vi "MPU_Stick_Read_Serial_Port.vi"(8 "error in (no error)":errorcluster, 11 "MPU_Stick_Globals":T1) -> ()   [LabVIEW 2017]
uses:
  Controls/MPU_Stick_Globals.ctl
  Controls/IMU_Configuration_References.ctl
  Controls/MP_Comp_Filter_Constants_References.ctl
  Controls/MD_Threshold_References.ctl
  Controls/MD_Type_References.ctl
  Controls/LED_Configuration_References.ctl
  Controls/Primary_References.ctl
  Controls/MPU_Stick_Queues.ctl
  Controls/MPU_Stick_Queue_Element.ctl
  Controls/MPU_Stick_Queue_Commands.ctl
  Classes/ADCP.lvclass
  Controls/MPU_Stick_Timestamped_Data.ctl
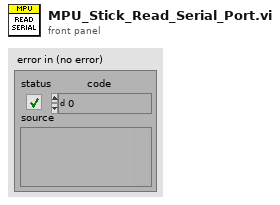
[diagram p1: front panel]
types:
  T1 = typedef "MPU_Stick_Globals.ctl" = cluster{"IMU_configuration_references":T2, "MP_Comp_Filter_Constants_References":T3, "MD_Threshold_References":T4, "MD_Type_References":T5, "LED_Configuration_References":T6, "Primary_references":T7, "MPU_Stick_Queues":T8, "ADCP":refnum<vi>}
  T2 = typedef "IMU_Configuration_References.ctl" = cluster{"Get all IMU configurations":refnum<vi>, "Set all IMU configurations":refnum<vi>, "Get sampling frequency":refnum<vi>, "Set sampling frequency":refnum<vi>, "Get calibration point count":refnum<vi>, "Set calibration point count":refnum<vi>, "Get calibration interval":refnum<vi>, "Set calibration interval":refnum<vi>, "Get Gyroscope bandwidth":refnum<vi>, "Set Gyroscope bandwidth":refnum<vi>, "Get Gyroscope F.S. Value":refnum<vi>, "Set Gyroscope F.S. Value":refnum<vi>, "Get Accelerometer bandwidth":refnum<vi>, "Set Accelerometer bandwidth":refnum<vi>, "Get Accelerometer F.S. Value":refnum<vi>, "Set Accelerometer F.S. Value":refnum<vi>, "Sampling frequency (Hz)":refnum<vi>, "Calibration point count":refnum<vi>, "Calibration interval (ms)":refnum<vi>, "IMU Gyroscope bandwidth":refnum<vi>, "IMU Gyroscope F.S. value":refnum<vi>, "IMU Accelerometer bandwidth":refnum<vi>, "IMU Accelerometer F.S. value":refnum<vi>}
  T3 = typedef "MP_Comp_Filter_Constants_References.ctl" = cluster{"Set pitch filter constant":refnum<vi>, "Get pitch filter constant":refnum<vi>, "Set roll filter constant":refnum<vi>, "Get roll filter constant":refnum<vi>, "Pitch filter constant":refnum<vi>, "Roll filter constant":refnum<vi>}
  T4 = typedef "MD_Threshold_References.ctl" = cluster{"Yaw threshold (U)":refnum<vi>, "Yaw threshold (L)":refnum<vi>, "Pitch threshold (U)":refnum<vi>, "Pitch. threshold (L)":refnum<vi>, "Roll threshold (U)":refnum<vi>, "Roll threshold (L)":refnum<vi>, "Z gyro. threshold (U)":refnum<vi>, "Z gyro. threshold (L)":refnum<vi>, "Y gyro. threshold (U)":refnum<vi>, "Y gyro. threshold (L)":refnum<vi>, "X gyro. threshold (U)":refnum<vi>, "X gyro. threshold (L)":refnum<vi>, "Z accel. threshold (U)":refnum<vi>, "Z accel. threshold (L)":refnum<vi>, "Y accel. threshold (U)":refnum<vi>, "Y accel. threshold (L)":refnum<vi>, "X accel. threshold (U)":refnum<vi>, "X accel. threshold (L)":refnum<vi>, "Set all Motion detection threshold configurations":refnum<vi>, "Get yaw threshold (upper)":refnum<vi>, "Get yaw threshold (lower)":refnum<vi>, "Get pitch threshold (upper)":refnum<vi>, "Get pitch threshold (lower)":refnum<vi>, "Get roll threshold (upper)":refnum<vi>, "Get roll threshold (lower)":refnum<vi>, "Get Z gyro threshold (upper)":refnum<vi>, "Get Z gyro threshold (lower)":refnum<vi>, "Get Y gyro threshold (upper)":refnum<vi>, "Get Y gyro threshold (lower)":refnum<vi>, "Get X gyro threshold (upper)":refnum<vi>, "Get X gyro threshold (lower)":refnum<vi>, "Get Z accel threshold (upper)":refnum<vi>, "Get Z accel threshold (lower)":refnum<vi>, "Get Y accel threshold (upper)":refnum<vi>, "Get Y accel threshold (lower)":refnum<vi>, "Get X accel threshold (upper)":refnum<vi>, "Get X accel threshold (lower)":refnum<vi>, "Get all Motion detection threshold configurations":refnum<vi>, "Set yaw threshold (upper)":refnum<vi>, "Set yaw threshold (lower)":refnum<vi>, "Set pitch threshold (upper)":refnum<vi>, "Set pitch threshold (lower)":refnum<vi>, "Set roll threshold (upper)":refnum<vi>, "Set roll threshold (lower)":refnum<vi>, "Set Z gyro threshold (upper)":refnum<vi>, "Set Z gyro threshold (lower)":refnum<vi>, "Set Y gyro threshold (upper)":refnum<vi>, "Set Y gyro threshold (lower)":refnum<vi>, "Set X gyro threshold (upper)":refnum<vi>, "Set X gyro threshold (lower)":refnum<vi>, "Set Z accel threshold (upper)":refnum<vi>, "Set Z accel threshold (lower)":refnum<vi>, "Set Y accel threshold (upper)":refnum<vi>, "Set Y accel threshold (lower)":refnum<vi>, "Set X accel threshold (upper)":refnum<vi>, "Set X accel threshold (lower)":refnum<vi>}
  T5 = typedef "MD_Type_References.ctl" = cluster{"Yaw threshold type":refnum<vi>, "Pitch threshold type":refnum<vi>, "Roll threshold type":refnum<vi>, "Z gyro threshold type":refnum<vi>, "Y gyro threshold type":refnum<vi>, "X gyro threshold type":refnum<vi>, "Z accel threshold type":refnum<vi>, "Y accel threshold type":refnum<vi>, "X accel threshold type":refnum<vi>, "Set all Motion detection type configurations":refnum<vi>, "Get all Motion detection type configurations":refnum<vi>, "Set yaw threshold type":refnum<vi>, "Get yaw threshold type":refnum<vi>, "Set pitch threshold type":refnum<vi>, "Get pitch threshold type":refnum<vi>, "Set roll threshold type":refnum<vi>, "Get roll threshold type":refnum<vi>, "Set Z gyroscope threshold type":refnum<vi>, "Get Z gyroscope threshold type":refnum<vi>, "Set Y gyroscope threshold type":refnum<vi>, "Get Y gyroscope threshold type":refnum<vi>, "Set X gyroscope threshold type":refnum<vi>, "Get X gyroscope threshold type":refnum<vi>, "Set Z accel threshold type":refnum<vi>, "Get Z accel threshold type":refnum<vi>, "Set Y accel threshold type":refnum<vi>, "Get Y accel threshold type":refnum<vi>, "Get X accel threshold type":refnum<vi>, "Set X accel threshold type":refnum<vi>}
  T6 = typedef "LED_Configuration_References.ctl" = cluster{"Get all LED configurations":refnum<vi>, "Set all LED configurations":refnum<vi>, "Get LED3 configuration":refnum<vi>, "Set LED3 configuration":refnum<vi>, "Get LED2 configuration":refnum<vi>, "Set LED2 configuration":refnum<vi>, "Get LED1 configuration":refnum<vi>, "Set LED1 configuration":refnum<vi>, "LED3 Configuration":refnum<vi>, "LED2 Configuration":refnum<vi>, "LED1 Configuration":refnum<vi>}
  T7 = typedef "Primary_References.ctl" = cluster{"3D View Image":refnum<vi>, "Plot":refnum<vi>, "Graph / 3D view tab control":refnum<vi>, "MP Reset":refnum<vi>, "Calibrate IMU":refnum<vi>, "Plot Parameter List":refnum<vi>, "Remove Parameter from Plot":refnum<vi>, "Add Parameter to Plot":refnum<vi>, "Parameter to monitor":refnum<vi>, "Yaw motion detection output":refnum<vi>, "Pitch motion detection output":refnum<vi>, "Roll motion detection output":refnum<vi>, "Z gyro motion detection output":refnum<vi>, "Y gyro motion detection output":refnum<vi>, "X gyro motion detection output":refnum<vi>, "Z accel motion detection output":refnum<vi>, "Y accel motion detection output":refnum<vi>, "X accel motion detection output":refnum<vi>, "Yaw angle (filter) (degrees)":refnum<vi>, "Pitch angle (filter) (degrees)":refnum<vi>, "Roll angle (filter) (degrees)":refnum<vi>, "Yaw angle (gyro) (degrees)":refnum<vi>, "Pitch angle (gyro) (degrees)":refnum<vi>, "Roll angle (gyro) (degrees)":refnum<vi>, "Yaw angle (accel) (degrees)":refnum<vi>, "Pitch angle (accel) (degrees)":refnum<vi>, "Roll angle (accel) (degrees)":refnum<vi>, "Z gyroscope reading (DPS)":refnum<vi>, "Y gyroscope reading (DPS)":refnum<vi>, "X gyroscope reading (DPS)":refnum<vi>, "Z accelerometer reading (G)":refnum<vi>, "Y accelerometer reading (G)":refnum<vi>, "X accelerometer reading (G)":refnum<vi>, "Save all config.":refnum<vi>, "Write all config.":refnum<vi>, "Read all config.":refnum<vi>, "Tab Control":refnum<vi>, "Baud Rate":refnum<vi>, "COM Port":refnum<vi>, "Time (ms)":refnum<vi>, "Value (Units)":refnum<vi>, "Exit Application":refnum<vi>, "Connect Device":refnum<vi>, "Progress Bar":refnum<vi>, "Get Range & Offset":refnum<vi>, "Range":refnum<vi>, "Offset":refnum<vi>, "Set Range & Offset":refnum<vi>, "Parameter name":refnum<vi>, "Plot time (ms)":refnum<vi>, "Plot value":refnum<vi>}
  T8 = typedef "MPU_Stick_Queues.ctl" = cluster{"UI Event Handler":refnum<queue>, "3D View Updater":refnum<queue>, "Plot Updater":refnum<queue>, "Serial Port Reader":refnum<queue>, "UI Indicators Updater":refnum<queue>}
  T9 = typedef "MPU_Stick_Queue_Commands.ctl" = enum16{"UI_Event_Exit_Application_RQST", "UI_Event_Exit_Application_ACK", "UI_Event_Connect_Device_RQST", "UI_Event_Connect_Device_ACK", "UI_Event_Disconnect_Device_RQST", "UI_Event_Disconnect_Device_ACK", "UI_Event_Read_All_Configurations_RQST", "UI_Event_Read_All_Configurations_ACK", "UI_Event_Write_All_Configurations_RQST", "UI_Event_Write_All_Configurations_ACK", "UI_Event_Save_All_Configurations_RQST", "UI_Event_Save_All_Configurations_ACK", "UI_Event_Calibrate_IMU_Sensor_RQST", "UI_Event_Calibrate_IMU_Sensor_ACK", "UI_Event_MP_Reset_RQST", "UI_Event_MP_Reset_ACK", "UI_Event_Get_Config_RQST", "UI_Event_Get_Config_ACK", "UI_Event_Set_Config_RQST", "UI_Event_Set_Config_ACK", "Read_Serial_Port_Data_Pause", "Read_Serial_Port_Data_Continue", "Read_Serial_Port_Data_Exit", "Plotter_Exit", "Plotter_Update", "Plotter_Add_Channel", "Plotter_Remove_Channel", "3D Viewer Update", "3D Viewer Exit", "UI Indicators Update", "UI Indicators Exit"}
  T10 = typedef "MPU_Stick_Queue_Element.ctl" = cluster{"Data":variant, "Command":T9}
  T11 = typedef "MPU_Stick_Timestamped_Data.ctl" = cluster{"Parameter name":string, "Time (ms)":dbl, "Value":dbl}
  T12 = typedef "ADCP.lvclass/ADCP_Packet_Info.ctl" = cluster{"Priority":enum16{"LOW", "HIGH"}, "Type":enum16{"Data", "Connection Management", "Remote Request", "Error and status", "INVALID"}, "Node ID":i32, "Frame ID":i32, "Checksum valid ?":bool, "Current time (ms)":u32}
  T13 = typedef "ADCP.lvclass/ADCP_Data_Packet_Transmit_Mode.ctl" = enum16{"Disable", "Single", "Cyclic", "Repeat"}
  T14 = cluster{"Parameters":cluster{"Parameter name":string, "Node name":string, "Node ID":u8, "Frame name":string, "Frame ID":u8, "Start bit":u32, "Bit length":u32, "Factor":dbl, "Offset":dbl, "Minimum":dbl, "Maximum":dbl, "Value":string, "Comments":string, "Data_Type":enum16{"BOOL", "UNSIGNED", "SIGNED", "FLOAT32", "ENUM"}, "Enum List":string[]}[], "Priority":enum16{"LOW", "HIGH"}, "Node name":string, "Node ID":u8, "Frame name":string, "Frame ID":u8, "Data":u32, "Raw bytes":u8[], "Processed bytes":u8[], "Tx count":i32, "Last Tx Time":u32, "Tx interval":u32, "Rx count":i32, "Last Rx Time":u32, "Rx interval":u32, "Tx Enable":bool, "Tx mode":T13, "Repeat/Cyclic Tx interval":u32, "Repeat count":u16}
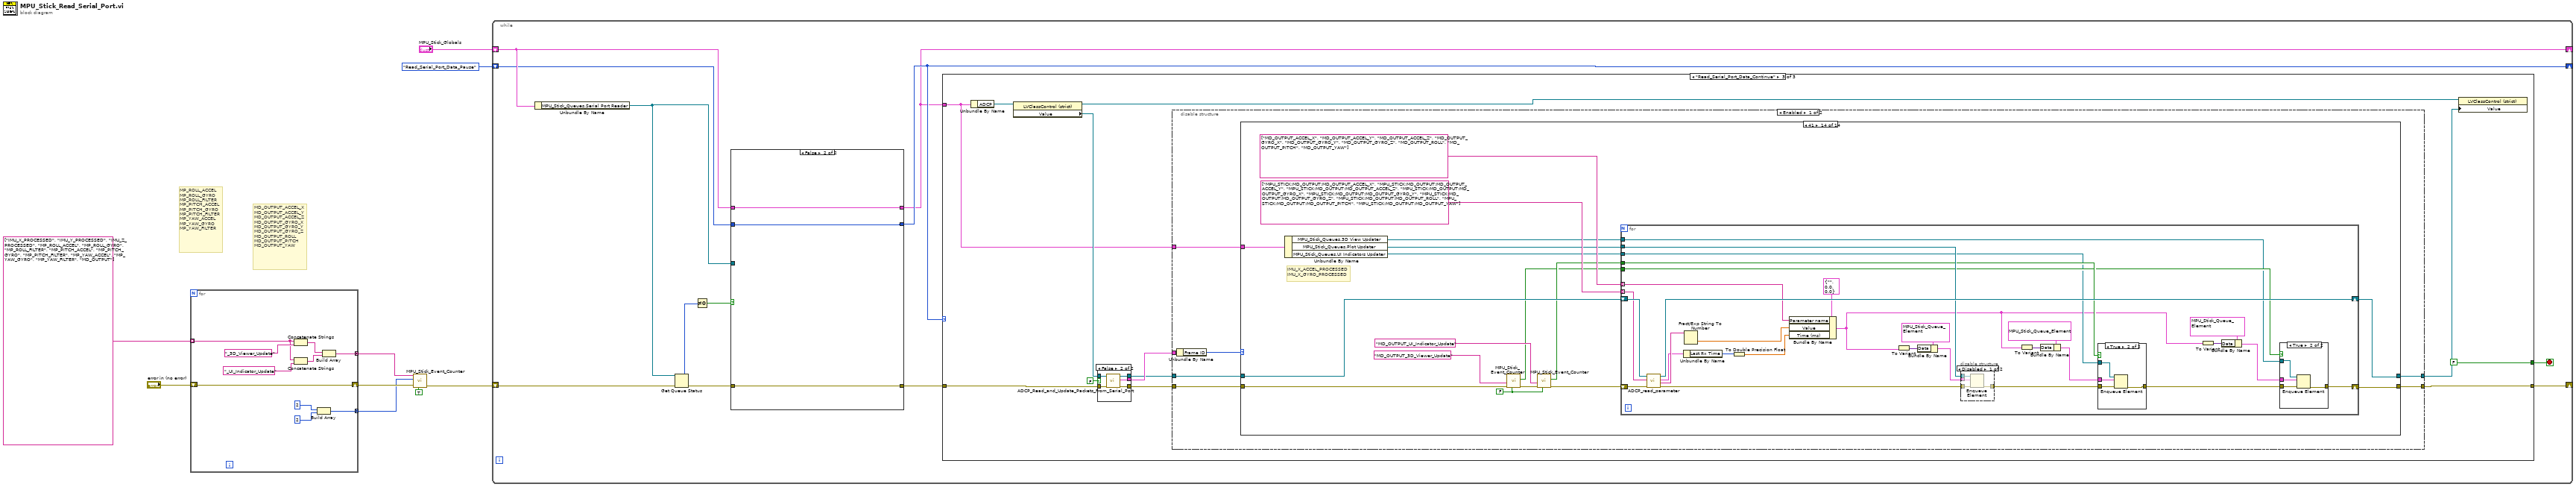
[diagram p0: block diagram]
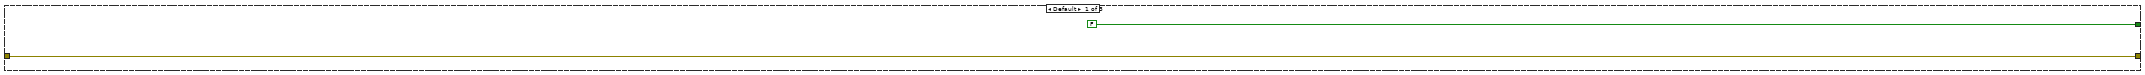
[diagram p2: hidden frame]
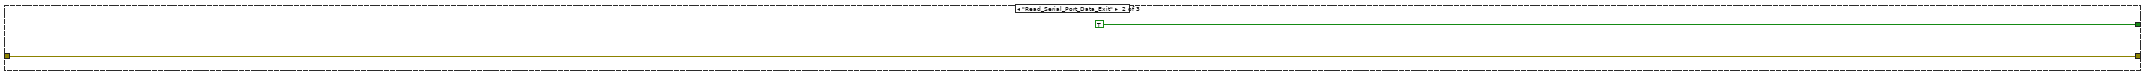
[diagram p3: hidden frame]
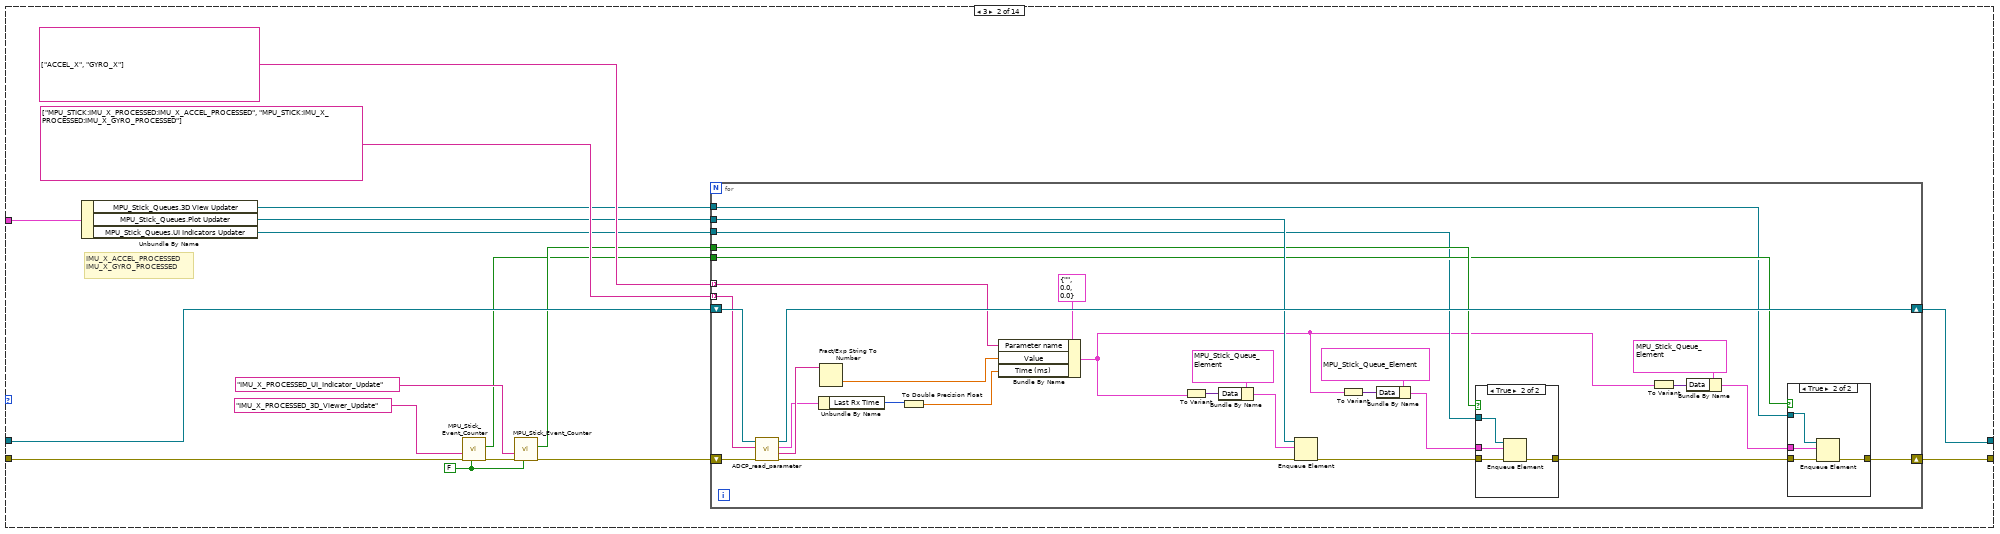
[diagram p5: hidden frame]
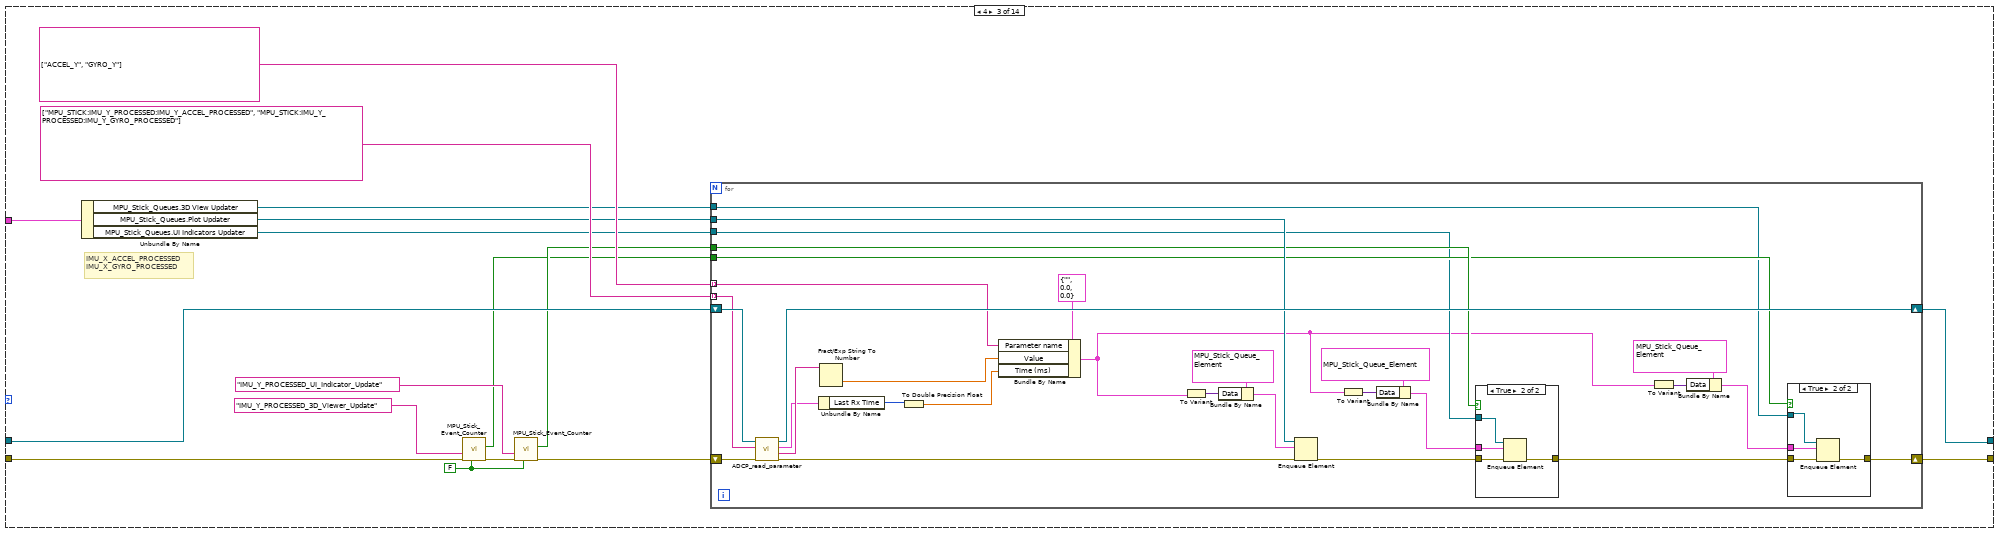
[diagram p8: hidden frame]
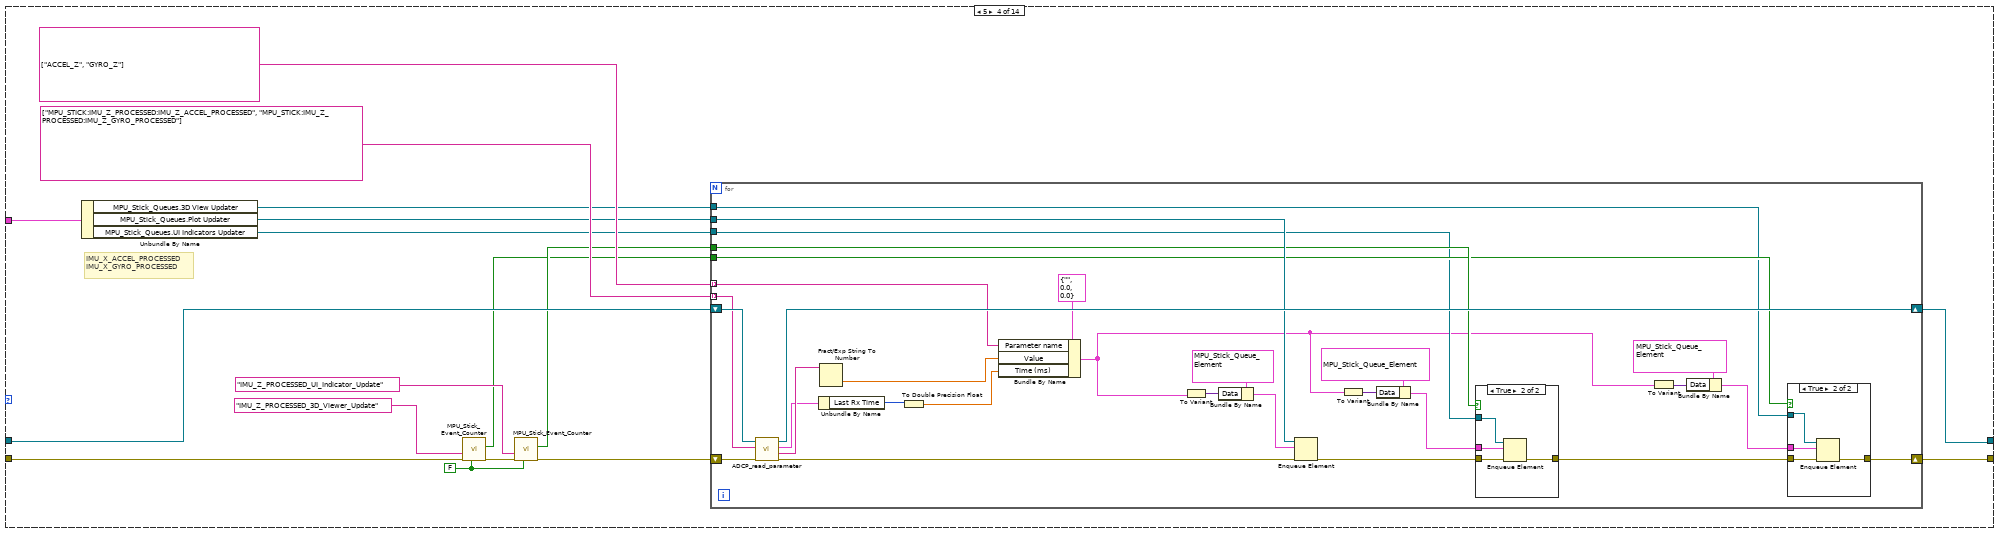
[diagram p11: hidden frame]
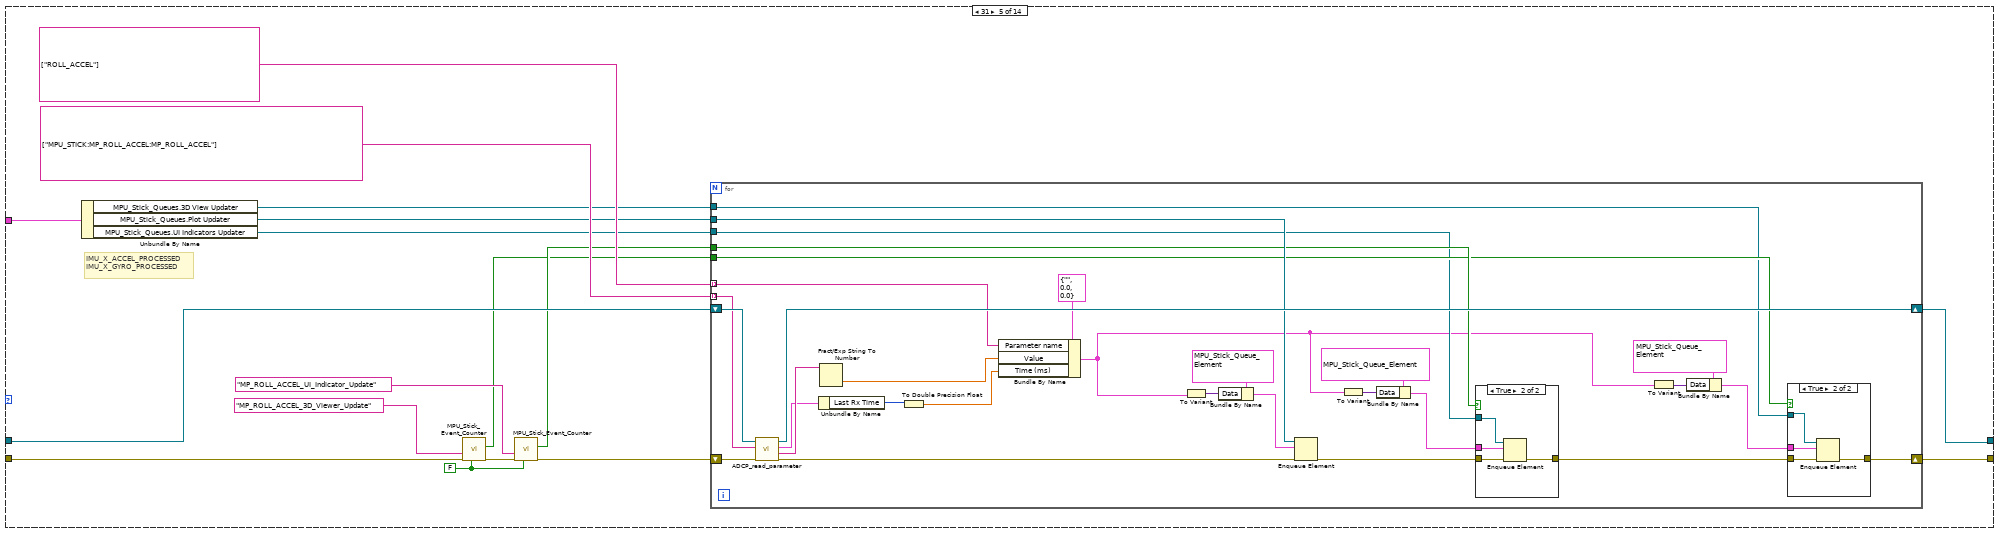
[diagram p14: hidden frame]
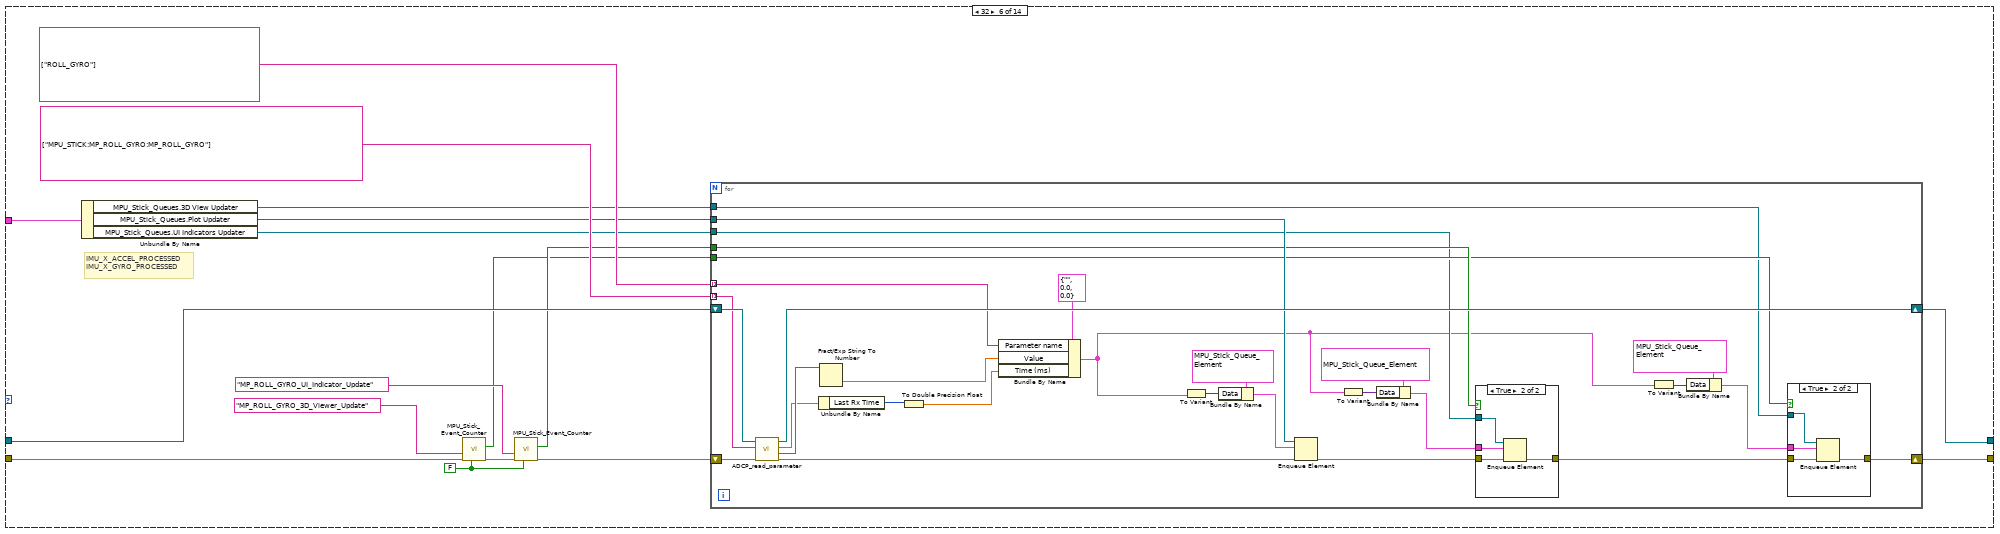
[diagram p17: hidden frame]
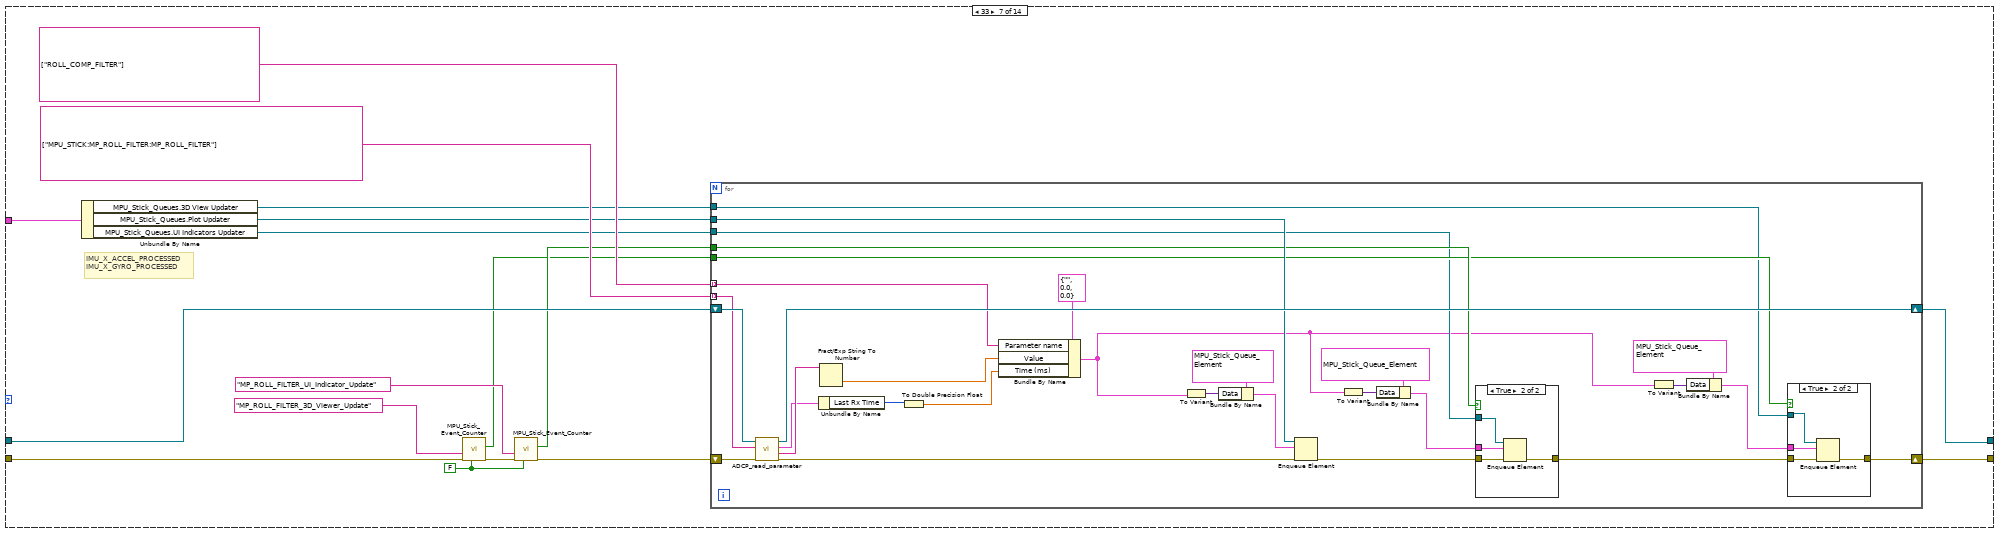
[diagram p20: hidden frame]
diagram:
  # "MD_OUTPUT_ACCEL_X\nMD_OUTPUT_ACCEL_Y\nMD_OUTPUT_ACCEL_Z\nMD_OUTPUT_GYRO_X\nMD_OUTPUT_GYRO_Y\nMD_OUTPUT_GYRO_Z\nMD_OUTPUT_ROLL\nMD_OUTPUT_PITCH\nMD_OUTPUT_YAW"
  # "MP_ROLL_ACCEL\nMP_ROLL_GYRO\nMP_ROLL_FILTER\nMP_PITCH_ACCEL\nMP_PITCH_GYRO\nMP_PITCH_FILTER\nMP_YAW_ACCEL\nMP_YAW_GYRO\nMP_YAW_FILTER"
  n1 = for {
    shift-right: [w19] -> w4
    shift-left: "error in (no error)" -> [w19]
    tunnel: [w14] -> w5 mode=concatenating
    tunnel: [w11] -> w3 mode=concatenating
    tunnel: string[] ["IMU_X_PROCESSED", "IMU_Y_PROCESSED", "IMU_Z_PROCESSED", "MP_ROLL_ACCEL", "MP_ROLL_GYRO", "MP_ROLL_FILTER", "MP_PITCH_ACCEL", "MP_PITCH_GYRO", "MP_PITCH_FILTER", "MP_YAW_ACCEL", "MP_YAW_GYRO", "MP_YAW_FILTER", "MD_OUTPUT"] -> [w10] mode=indexing
    n2 = Concatenate Strings(w10, "_3D_Viewer_Update" ("string")) -> (w16:string)
    n3 = Concatenate Strings(w10, "_UI_Indicator_Update" ("string")) -> (w15:string)
    n4 = Build Array(2, 2) -> (w11:i32[])
    n5 = Build Array(w16, w15) -> (w14:string[])
  }
  n6 = call "MPU_Stick_Event_Counter.vi"("Initialize ?"=TRUE, "error in (no error)"=w4, "Event count limits"=w3, "Event names"=w5) -> ("error out"=w7:errorcluster)  [unwired: 5 in, 2 out]
  n7 = while {
    shift-right: [w22] -> _
    shift-left: w7 -> [w31]
    shift-right: [w20] -> _
    shift-left: "MPU_Stick_Globals" -> [w27]
    shift-right: [w23] -> _
    shift-left: MPU_Stick_Queue_Commands."Read_Serial_Port_Data_Pause" ("Command") -> [w25]
    stop <- w21 stop-if-true
    n8 = Unbundle By Name(w27) -> ("MPU_Stick_Queues.Serial Port Reader"=w26:refnum<queue>)
    n9 = Get Queue Status(queue=w26, error in (no error)=w31) -> (error out=w28:errorcluster, # elements in queue=w30:i32)  [unwired: 1 in, 6 out]
    n10 = Not Equal To 0?(x=w30) -> (x != 0?=w29:bool)
    n11 = case shown="False" w29 {
      tunnel: w28 -> [w819 w822]
      tunnel: w27 -> [w820 w823]
      tunnel: [w817 w822] -> w24
      tunnel: [w820 w823] -> w20
      tunnel: w26 -> [w818 _]
      tunnel: [w815 w821] -> w23
      tunnel: w25 -> [_ w821]
      frame True {
        n12 = Dequeue Element(queue=w818, error in (no error)=w819) -> (element=w816:T10, error out=w817:errorcluster)  [unwired: 1 in, 2 out]
        n13 = Unbundle By Name(w816) -> ("Command"=w815:T9)
      }
      frame False {
      }
    }
    n14 = case shown="\"Read_Serial_Port_Data_Continue\"" w23 {
      tunnel: w24 -> [w33 w35 w45]
      tunnel: [w33 w35 w38] -> w22
      tunnel: [FALSE TRUE FALSE] -> w21
      tunnel: w20 -> [_ _ w37]
      frame Default {
      }
      frame "Read_Serial_Port_Data_Exit" {
      }
      frame "Read_Serial_Port_Data_Continue" {
        n15 = Unbundle By Name(w37) -> ("ADCP"=w46:refnum<vi>)
        n16 = property class="LVClassControl (strict)"(reference=w46) -> (reference out=w43:refnum<vi>, "Value"=w44:refnum<class "ADCP.lvclass">)  [unwired: 1 in, 1 out]
        n17 = case shown="False" FALSE {
          tunnel: w45 -> [w806 w814]
          tunnel: w44 -> [w808 w813]
          tunnel: [w809 w812] -> w42
          tunnel: [w805 w811] -> w41
          tunnel: [w807 w810] -> w40
          frame True {
            n18 = call "ADCP_Read_and_Update_Packets_From_Serial_Port_Emulator.vi"("error in (no error)"=w806, "ADCP In"=w808) -> ("error out"=w805:errorcluster, "Packet Info"=w809:T12, "ADCP out"=w807:refnum<class "ADCP.lvclass">)  [unwired: 6 in, 1 out]
          }
          frame False {
            n19 = call "ADCP_Read_and_Update_Packets_From_Serial_Port.vi"("error in (no error)"=w814, "ADCP In"=w813) -> ("error out"=w811:errorcluster, "Packet Info"=w812:T12, "ADCP out"=w810:refnum<class "ADCP.lvclass">)  [unwired: 6 in, 1 out]
          }
        }
        n20 = disable-structure shown="Enabled" {
          disable-tunnel: w42 -> [w54 _]
          disable-tunnel: w41 -> [w52 w804]
          disable-tunnel: w40 -> [w51 w803]
          disable-tunnel: [w50 w803] -> w39
          disable-tunnel: [w49 w804] -> w38
          disable-tunnel: w37 -> [w48 _]
          frame Enabled {
            n21 = Unbundle By Name(w54) -> ("Frame ID"=w53:i32)
            n22 = case shown="41" w53 {
              tunnel: w52 -> [w55 w64 w121 w178 w235 w292 w349 w406 w463 w520 w577 w634 w691 w748]
              tunnel: w51 -> [w56 w73 w130 w187 w244 w301 w358 w415 w472 w529 w586 w643 w700 w757]
              tunnel: [w56 w71 w128 w185 w242 w299 w356 w413 w470 w527 w584 w641 w698 w755] -> w50
              tunnel: [w55 w68 w125 w182 w239 w296 w353 w410 w467 w524 w581 w638 w695 w752] -> w49
              tunnel: w48 -> [_ w70 w127 w184 w241 w298 w355 w412 w469 w526 w583 w640 w697 w754]
              frame Default {
              }
              frame 3 {
                w61 = FALSE ("Initialize ?")
                # "IMU_X_ACCEL_PROCESSED\nIMU_X_GYRO_PROCESSED"
                n23 = Unbundle By Name(w70) -> ("MPU_Stick_Queues.3D View Updater"=w67:refnum<queue>, "MPU_Stick_Queues.Plot Updater"=w66:refnum<queue>, "MPU_Stick_Queues.UI Indicators Updater"=w65:refnum<queue>)
                n24 = call "MPU_Stick_Event_Counter.vi"("Initialize ?"=w61, "error in (no error)"=w64, "Event Name"="IMU_X_PROCESSED_3D_Viewer_Update") -> ("error out"=w63:errorcluster, "Event occured"=w57:bool)  [unwired: 6 in, 1 out]
                n25 = call "MPU_Stick_Event_Counter.vi"("Initialize ?"=w61, "error in (no error)"=w63, "Event Name"="IMU_X_PROCESSED_UI_Indicator_Update") -> ("error out"=w62:errorcluster, "Event occured"=w58:bool)  [unwired: 6 in, 1 out]
                n26 = for {
                  shift-right: [w101] -> w71
                  shift-left: w73 -> [w103]
                  tunnel: string[] ["ACCEL_X", "GYRO_X"] -> [w95] mode=indexing
                  shift-right: [w84] -> w68
                  shift-left: w62 -> [w102]
                  tunnel: string[] ["MPU_STICK:IMU_X_PROCESSED:IMU_X_ACCEL_PROCESSED", "MPU_STICK:IMU_X_PROCESSED:IMU_X_GYRO_PROCESSED"] -> [w98] mode=indexing
                  tunnel: w67 -> [w82]
                  tunnel: w66 -> [w91]
                  tunnel: w65 -> [w83]
                  tunnel: w58 -> [w87]
                  tunnel: w57 -> [w85]
                  n27 = call "ADCP_read_parameter.vi"("error in (no error)"=w102, "Parameter Name"=w98, "ADCP In"=w103) -> ("error out"=w92:errorcluster, "Parameter Value"=w100:string, "Data Packet out"=w99:T14, "ADCP out"=w101:refnum<class "ADCP.lvclass">)  [unwired: 5 in]
                  n28 = Unbundle By Name(w99) -> ("Last Rx Time"=w97:u32)
                  n29 = Fract/Exp String To Number(string=w100) -> (number=w94:dbl)  [unwired: 3 in, 1 out]
                  n30 = To Double Precision Float(number=w97) -> (double precision float=w93:dbl)
                  n31 = Bundle By Name(cluster=T11 {"Parameter name"="", "Time (ms)"=0.0, "Value"=0.0}, "Parameter name"=w95, "Value"=w94, "Time (ms)"=w93) -> (w75:T11)
                  n32 = To Variant(anything=w75) -> (Variant=w89:variant)
                  n33 = Bundle By Name(cluster=T10 {"Data"=variant, "Command"=enum."Plotter_Update"} ("element"), "Data"=w89) -> (w81:T10)
                  n34 = Enqueue Element(queue=w91, element=w81, error in (no error)=w92) -> (error out=w88:errorcluster)  [unwired: 1 in, 2 out]
                  n35 = To Variant(anything=w75) -> (Variant=w79:variant)
                  n36 = Bundle By Name(cluster=T10 {"Data"=variant, "Command"=enum."UI Indicators Update"} ("element"), "Data"=w79) -> (w78:T10)
                  n37 = case shown="True" w87 {
                    tunnel: w88 -> [w109 w113]
                    tunnel: [w109 w111] -> w86
                    tunnel: w83 -> [_ w112]
                    tunnel: w78 -> [_ w110]
                    frame False {
                    }
                    frame True {
                      n38 = Enqueue Element(queue=w112, element=w110, error in (no error)=w113) -> (error out=w111:errorcluster)  [unwired: 1 in, 2 out]
                    }
                  }
                  n39 = To Variant(anything=w75) -> (Variant=w76:variant)
                  n40 = Bundle By Name(cluster=T10 {"Data"=variant, "Command"=enum."3D Viewer Update"} ("element"), "Data"=w76) -> (w74:T10)
                  n41 = case shown="True" w85 {
                    tunnel: w86 -> [w104 w108]
                    tunnel: [w104 w105] -> w84
                    tunnel: w82 -> [_ w107]
                    tunnel: w74 -> [_ w106]
                    frame False {
                    }
                    frame True {
                      n42 = Enqueue Element(queue=w107, element=w106, error in (no error)=w108) -> (error out=w105:errorcluster)  [unwired: 1 in, 2 out]
                    }
                  }
                }
              }
              frame 4 {
                w118 = FALSE ("Initialize ?")
                # "IMU_X_ACCEL_PROCESSED\nIMU_X_GYRO_PROCESSED"
                n43 = Unbundle By Name(w127) -> ("MPU_Stick_Queues.3D View Updater"=w124:refnum<queue>, "MPU_Stick_Queues.Plot Updater"=w123:refnum<queue>, "MPU_Stick_Queues.UI Indicators Updater"=w122:refnum<queue>)
                n44 = call "MPU_Stick_Event_Counter.vi"("Initialize ?"=w118, "error in (no error)"=w121, "Event Name"="IMU_Y_PROCESSED_3D_Viewer_Update") -> ("error out"=w120:errorcluster, "Event occured"=w114:bool)  [unwired: 6 in, 1 out]
                n45 = call "MPU_Stick_Event_Counter.vi"("Initialize ?"=w118, "error in (no error)"=w120, "Event Name"="IMU_Y_PROCESSED_UI_Indicator_Update") -> ("error out"=w119:errorcluster, "Event occured"=w115:bool)  [unwired: 6 in, 1 out]
                n46 = for {
                  shift-right: [w158] -> w128
                  shift-left: w130 -> [w160]
                  tunnel: string[] ["ACCEL_Y", "GYRO_Y"] -> [w152] mode=indexing
                  shift-right: [w141] -> w125
                  shift-left: w119 -> [w159]
                  tunnel: string[] ["MPU_STICK:IMU_Y_PROCESSED:IMU_Y_ACCEL_PROCESSED", "MPU_STICK:IMU_Y_PROCESSED:IMU_Y_GYRO_PROCESSED"] -> [w155] mode=indexing
                  tunnel: w124 -> [w139]
                  tunnel: w123 -> [w148]
                  tunnel: w122 -> [w140]
                  tunnel: w115 -> [w144]
                  tunnel: w114 -> [w142]
                  n47 = call "ADCP_read_parameter.vi"("error in (no error)"=w159, "Parameter Name"=w155, "ADCP In"=w160) -> ("error out"=w149:errorcluster, "Parameter Value"=w157:string, "Data Packet out"=w156:T14, "ADCP out"=w158:refnum<class "ADCP.lvclass">)  [unwired: 5 in]
                  n48 = Unbundle By Name(w156) -> ("Last Rx Time"=w154:u32)
                  n49 = Fract/Exp String To Number(string=w157) -> (number=w151:dbl)  [unwired: 3 in, 1 out]
                  n50 = To Double Precision Float(number=w154) -> (double precision float=w150:dbl)
                  n51 = Bundle By Name(cluster=T11 {"Parameter name"="", "Time (ms)"=0.0, "Value"=0.0}, "Parameter name"=w152, "Value"=w151, "Time (ms)"=w150) -> (w132:T11)
                  n52 = To Variant(anything=w132) -> (Variant=w146:variant)
                  n53 = Bundle By Name(cluster=T10 {"Data"=variant, "Command"=enum."Plotter_Update"} ("element"), "Data"=w146) -> (w138:T10)
                  n54 = Enqueue Element(queue=w148, element=w138, error in (no error)=w149) -> (error out=w145:errorcluster)  [unwired: 1 in, 2 out]
                  n55 = To Variant(anything=w132) -> (Variant=w136:variant)
                  n56 = Bundle By Name(cluster=T10 {"Data"=variant, "Command"=enum."UI Indicators Update"} ("element"), "Data"=w136) -> (w135:T10)
                  n57 = case shown="True" w144 {
                    tunnel: w145 -> [w166 w170]
                    tunnel: [w166 w168] -> w143
                    tunnel: w140 -> [_ w169]
                    tunnel: w135 -> [_ w167]
                    frame False {
                    }
                    frame True {
                      n58 = Enqueue Element(queue=w169, element=w167, error in (no error)=w170) -> (error out=w168:errorcluster)  [unwired: 1 in, 2 out]
                    }
                  }
                  n59 = To Variant(anything=w132) -> (Variant=w133:variant)
                  n60 = Bundle By Name(cluster=T10 {"Data"=variant, "Command"=enum."3D Viewer Update"} ("element"), "Data"=w133) -> (w131:T10)
                  n61 = case shown="True" w142 {
                    tunnel: w143 -> [w161 w165]
                    tunnel: [w161 w162] -> w141
                    tunnel: w139 -> [_ w164]
                    tunnel: w131 -> [_ w163]
                    frame False {
                    }
                    frame True {
                      n62 = Enqueue Element(queue=w164, element=w163, error in (no error)=w165) -> (error out=w162:errorcluster)  [unwired: 1 in, 2 out]
                    }
                  }
                }
              }
              frame 5 {
                w175 = FALSE ("Initialize ?")
                # "IMU_X_ACCEL_PROCESSED\nIMU_X_GYRO_PROCESSED"
                n63 = Unbundle By Name(w184) -> ("MPU_Stick_Queues.3D View Updater"=w181:refnum<queue>, "MPU_Stick_Queues.Plot Updater"=w180:refnum<queue>, "MPU_Stick_Queues.UI Indicators Updater"=w179:refnum<queue>)
                n64 = call "MPU_Stick_Event_Counter.vi"("Initialize ?"=w175, "error in (no error)"=w178, "Event Name"="IMU_Z_PROCESSED_3D_Viewer_Update") -> ("error out"=w177:errorcluster, "Event occured"=w171:bool)  [unwired: 6 in, 1 out]
                n65 = call "MPU_Stick_Event_Counter.vi"("Initialize ?"=w175, "error in (no error)"=w177, "Event Name"="IMU_Z_PROCESSED_UI_Indicator_Update") -> ("error out"=w176:errorcluster, "Event occured"=w172:bool)  [unwired: 6 in, 1 out]
                n66 = for {
                  shift-right: [w215] -> w185
                  shift-left: w187 -> [w217]
                  tunnel: string[] ["ACCEL_Z", "GYRO_Z"] -> [w209] mode=indexing
                  shift-right: [w198] -> w182
                  shift-left: w176 -> [w216]
                  tunnel: string[] ["MPU_STICK:IMU_Z_PROCESSED:IMU_Z_ACCEL_PROCESSED", "MPU_STICK:IMU_Z_PROCESSED:IMU_Z_GYRO_PROCESSED"] -> [w212] mode=indexing
                  tunnel: w181 -> [w196]
                  tunnel: w180 -> [w205]
                  tunnel: w179 -> [w197]
                  tunnel: w172 -> [w201]
                  tunnel: w171 -> [w199]
                  n67 = call "ADCP_read_parameter.vi"("error in (no error)"=w216, "Parameter Name"=w212, "ADCP In"=w217) -> ("error out"=w206:errorcluster, "Parameter Value"=w214:string, "Data Packet out"=w213:T14, "ADCP out"=w215:refnum<class "ADCP.lvclass">)  [unwired: 5 in]
                  n68 = Unbundle By Name(w213) -> ("Last Rx Time"=w211:u32)
                  n69 = Fract/Exp String To Number(string=w214) -> (number=w208:dbl)  [unwired: 3 in, 1 out]
                  n70 = To Double Precision Float(number=w211) -> (double precision float=w207:dbl)
                  n71 = Bundle By Name(cluster=T11 {"Parameter name"="", "Time (ms)"=0.0, "Value"=0.0}, "Parameter name"=w209, "Value"=w208, "Time (ms)"=w207) -> (w189:T11)
                  n72 = To Variant(anything=w189) -> (Variant=w203:variant)
                  n73 = Bundle By Name(cluster=T10 {"Data"=variant, "Command"=enum."Plotter_Update"} ("element"), "Data"=w203) -> (w195:T10)
                  n74 = Enqueue Element(queue=w205, element=w195, error in (no error)=w206) -> (error out=w202:errorcluster)  [unwired: 1 in, 2 out]
                  n75 = To Variant(anything=w189) -> (Variant=w193:variant)
                  n76 = Bundle By Name(cluster=T10 {"Data"=variant, "Command"=enum."UI Indicators Update"} ("element"), "Data"=w193) -> (w192:T10)
                  n77 = case shown="True" w201 {
                    tunnel: w202 -> [w223 w227]
                    tunnel: [w223 w225] -> w200
                    tunnel: w197 -> [_ w226]
                    tunnel: w192 -> [_ w224]
                    frame False {
                    }
                    frame True {
                      n78 = Enqueue Element(queue=w226, element=w224, error in (no error)=w227) -> (error out=w225:errorcluster)  [unwired: 1 in, 2 out]
                    }
                  }
                  n79 = To Variant(anything=w189) -> (Variant=w190:variant)
                  n80 = Bundle By Name(cluster=T10 {"Data"=variant, "Command"=enum."3D Viewer Update"} ("element"), "Data"=w190) -> (w188:T10)
                  n81 = case shown="True" w199 {
                    tunnel: w200 -> [w218 w222]
                    tunnel: [w218 w219] -> w198
                    tunnel: w196 -> [_ w221]
                    tunnel: w188 -> [_ w220]
                    frame False {
                    }
                    frame True {
                      n82 = Enqueue Element(queue=w221, element=w220, error in (no error)=w222) -> (error out=w219:errorcluster)  [unwired: 1 in, 2 out]
                    }
                  }
                }
              }
              frame 31 {
                w232 = FALSE ("Initialize ?")
                # "IMU_X_ACCEL_PROCESSED\nIMU_X_GYRO_PROCESSED"
                n83 = Unbundle By Name(w241) -> ("MPU_Stick_Queues.3D View Updater"=w238:refnum<queue>, "MPU_Stick_Queues.Plot Updater"=w237:refnum<queue>, "MPU_Stick_Queues.UI Indicators Updater"=w236:refnum<queue>)
                n84 = call "MPU_Stick_Event_Counter.vi"("Initialize ?"=w232, "error in (no error)"=w235, "Event Name"="MP_ROLL_ACCEL_3D_Viewer_Update") -> ("error out"=w234:errorcluster, "Event occured"=w228:bool)  [unwired: 6 in, 1 out]
                n85 = call "MPU_Stick_Event_Counter.vi"("Initialize ?"=w232, "error in (no error)"=w234, "Event Name"="MP_ROLL_ACCEL_UI_Indicator_Update") -> ("error out"=w233:errorcluster, "Event occured"=w229:bool)  [unwired: 6 in, 1 out]
                n86 = for {
                  shift-right: [w272] -> w242
                  shift-left: w244 -> [w274]
                  tunnel: string[] ["ROLL_ACCEL"] -> [w266] mode=indexing
                  shift-right: [w255] -> w239
                  shift-left: w233 -> [w273]
                  tunnel: string[] ["MPU_STICK:MP_ROLL_ACCEL:MP_ROLL_ACCEL"] -> [w269] mode=indexing
                  tunnel: w238 -> [w253]
                  tunnel: w237 -> [w262]
                  tunnel: w236 -> [w254]
                  tunnel: w229 -> [w258]
                  tunnel: w228 -> [w256]
                  n87 = call "ADCP_read_parameter.vi"("error in (no error)"=w273, "Parameter Name"=w269, "ADCP In"=w274) -> ("error out"=w263:errorcluster, "Parameter Value"=w271:string, "Data Packet out"=w270:T14, "ADCP out"=w272:refnum<class "ADCP.lvclass">)  [unwired: 5 in]
                  n88 = Unbundle By Name(w270) -> ("Last Rx Time"=w268:u32)
                  n89 = Fract/Exp String To Number(string=w271) -> (number=w265:dbl)  [unwired: 3 in, 1 out]
                  n90 = To Double Precision Float(number=w268) -> (double precision float=w264:dbl)
                  n91 = Bundle By Name(cluster=T11 {"Parameter name"="", "Time (ms)"=0.0, "Value"=0.0}, "Parameter name"=w266, "Value"=w265, "Time (ms)"=w264) -> (w246:T11)
                  n92 = To Variant(anything=w246) -> (Variant=w260:variant)
                  n93 = Bundle By Name(cluster=T10 {"Data"=variant, "Command"=enum."Plotter_Update"} ("element"), "Data"=w260) -> (w252:T10)
                  n94 = Enqueue Element(queue=w262, element=w252, error in (no error)=w263) -> (error out=w259:errorcluster)  [unwired: 1 in, 2 out]
                  n95 = To Variant(anything=w246) -> (Variant=w250:variant)
                  n96 = Bundle By Name(cluster=T10 {"Data"=variant, "Command"=enum."UI Indicators Update"} ("element"), "Data"=w250) -> (w249:T10)
                  n97 = case shown="True" w258 {
                    tunnel: w259 -> [w280 w284]
                    tunnel: [w280 w282] -> w257
                    tunnel: w254 -> [_ w283]
                    tunnel: w249 -> [_ w281]
                    frame False {
                    }
                    frame True {
                      n98 = Enqueue Element(queue=w283, element=w281, error in (no error)=w284) -> (error out=w282:errorcluster)  [unwired: 1 in, 2 out]
                    }
                  }
                  n99 = To Variant(anything=w246) -> (Variant=w247:variant)
                  n100 = Bundle By Name(cluster=T10 {"Data"=variant, "Command"=enum."3D Viewer Update"} ("element"), "Data"=w247) -> (w245:T10)
                  n101 = case shown="True" w256 {
                    tunnel: w257 -> [w275 w279]
                    tunnel: [w275 w276] -> w255
                    tunnel: w253 -> [_ w278]
                    tunnel: w245 -> [_ w277]
                    frame False {
                    }
                    frame True {
                      n102 = Enqueue Element(queue=w278, element=w277, error in (no error)=w279) -> (error out=w276:errorcluster)  [unwired: 1 in, 2 out]
                    }
                  }
                }
              }
              frame 32 {
                w289 = FALSE ("Initialize ?")
                # "IMU_X_ACCEL_PROCESSED\nIMU_X_GYRO_PROCESSED"
                n103 = Unbundle By Name(w298) -> ("MPU_Stick_Queues.3D View Updater"=w295:refnum<queue>, "MPU_Stick_Queues.Plot Updater"=w294:refnum<queue>, "MPU_Stick_Queues.UI Indicators Updater"=w293:refnum<queue>)
                n104 = call "MPU_Stick_Event_Counter.vi"("Initialize ?"=w289, "error in (no error)"=w292, "Event Name"="MP_ROLL_GYRO_3D_Viewer_Update") -> ("error out"=w291:errorcluster, "Event occured"=w285:bool)  [unwired: 6 in, 1 out]
                n105 = call "MPU_Stick_Event_Counter.vi"("Initialize ?"=w289, "error in (no error)"=w291, "Event Name"="MP_ROLL_GYRO_UI_Indicator_Update") -> ("error out"=w290:errorcluster, "Event occured"=w286:bool)  [unwired: 6 in, 1 out]
                n106 = for {
                  shift-right: [w329] -> w299
                  shift-left: w301 -> [w331]
                  tunnel: string[] ["ROLL_GYRO"] -> [w323] mode=indexing
                  shift-right: [w312] -> w296
                  shift-left: w290 -> [w330]
                  tunnel: string[] ["MPU_STICK:MP_ROLL_GYRO:MP_ROLL_GYRO"] -> [w326] mode=indexing
                  tunnel: w295 -> [w310]
                  tunnel: w294 -> [w319]
                  tunnel: w293 -> [w311]
                  tunnel: w286 -> [w315]
                  tunnel: w285 -> [w313]
                  n107 = call "ADCP_read_parameter.vi"("error in (no error)"=w330, "Parameter Name"=w326, "ADCP In"=w331) -> ("error out"=w320:errorcluster, "Parameter Value"=w328:string, "Data Packet out"=w327:T14, "ADCP out"=w329:refnum<class "ADCP.lvclass">)  [unwired: 5 in]
                  n108 = Unbundle By Name(w327) -> ("Last Rx Time"=w325:u32)
                  n109 = Fract/Exp String To Number(string=w328) -> (number=w322:dbl)  [unwired: 3 in, 1 out]
                  n110 = To Double Precision Float(number=w325) -> (double precision float=w321:dbl)
                  n111 = Bundle By Name(cluster=T11 {"Parameter name"="", "Time (ms)"=0.0, "Value"=0.0}, "Parameter name"=w323, "Value"=w322, "Time (ms)"=w321) -> (w303:T11)
                  n112 = To Variant(anything=w303) -> (Variant=w317:variant)
                  n113 = Bundle By Name(cluster=T10 {"Data"=variant, "Command"=enum."Plotter_Update"} ("element"), "Data"=w317) -> (w309:T10)
                  n114 = Enqueue Element(queue=w319, element=w309, error in (no error)=w320) -> (error out=w316:errorcluster)  [unwired: 1 in, 2 out]
                  n115 = To Variant(anything=w303) -> (Variant=w307:variant)
                  n116 = Bundle By Name(cluster=T10 {"Data"=variant, "Command"=enum."UI Indicators Update"} ("element"), "Data"=w307) -> (w306:T10)
                  n117 = case shown="True" w315 {
                    tunnel: w316 -> [w337 w341]
                    tunnel: [w337 w339] -> w314
                    tunnel: w311 -> [_ w340]
                    tunnel: w306 -> [_ w338]
                    frame False {
                    }
                    frame True {
                      n118 = Enqueue Element(queue=w340, element=w338, error in (no error)=w341) -> (error out=w339:errorcluster)  [unwired: 1 in, 2 out]
                    }
                  }
                  n119 = To Variant(anything=w303) -> (Variant=w304:variant)
                  n120 = Bundle By Name(cluster=T10 {"Data"=variant, "Command"=enum."3D Viewer Update"} ("element"), "Data"=w304) -> (w302:T10)
                  n121 = case shown="True" w313 {
                    tunnel: w314 -> [w332 w336]
                    tunnel: [w332 w333] -> w312
                    tunnel: w310 -> [_ w335]
                    tunnel: w302 -> [_ w334]
                    frame False {
                    }
                    frame True {
                      n122 = Enqueue Element(queue=w335, element=w334, error in (no error)=w336) -> (error out=w333:errorcluster)  [unwired: 1 in, 2 out]
                    }
                  }
                }
              }
              frame 33 {
                w346 = FALSE ("Initialize ?")
                # "IMU_X_ACCEL_PROCESSED\nIMU_X_GYRO_PROCESSED"
                n123 = Unbundle By Name(w355) -> ("MPU_Stick_Queues.3D View Updater"=w352:refnum<queue>, "MPU_Stick_Queues.Plot Updater"=w351:refnum<queue>, "MPU_Stick_Queues.UI Indicators Updater"=w350:refnum<queue>)
                n124 = call "MPU_Stick_Event_Counter.vi"("Initialize ?"=w346, "error in (no error)"=w349, "Event Name"="MP_ROLL_FILTER_3D_Viewer_Update") -> ("error out"=w348:errorcluster, "Event occured"=w342:bool)  [unwired: 6 in, 1 out]
                n125 = call "MPU_Stick_Event_Counter.vi"("Initialize ?"=w346, "error in (no error)"=w348, "Event Name"="MP_ROLL_FILTER_UI_Indicator_Update") -> ("error out"=w347:errorcluster, "Event occured"=w343:bool)  [unwired: 6 in, 1 out]
                n126 = for {
                  shift-right: [w386] -> w356
                  shift-left: w358 -> [w388]
                  tunnel: string[] ["ROLL_COMP_FILTER"] -> [w380] mode=indexing
                  shift-right: [w369] -> w353
                  shift-left: w347 -> [w387]
                  tunnel: string[] ["MPU_STICK:MP_ROLL_FILTER:MP_ROLL_FILTER"] -> [w383] mode=indexing
                  tunnel: w352 -> [w367]
                  tunnel: w351 -> [w376]
                  tunnel: w350 -> [w368]
                  tunnel: w343 -> [w372]
                  tunnel: w342 -> [w370]
                  n127 = call "ADCP_read_parameter.vi"("error in (no error)"=w387, "Parameter Name"=w383, "ADCP In"=w388) -> ("error out"=w377:errorcluster, "Parameter Value"=w385:string, "Data Packet out"=w384:T14, "ADCP out"=w386:refnum<class "ADCP.lvclass">)  [unwired: 5 in]
                  n128 = Unbundle By Name(w384) -> ("Last Rx Time"=w382:u32)
                  n129 = Fract/Exp String To Number(string=w385) -> (number=w379:dbl)  [unwired: 3 in, 1 out]
                  n130 = To Double Precision Float(number=w382) -> (double precision float=w378:dbl)
                  n131 = Bundle By Name(cluster=T11 {"Parameter name"="", "Time (ms)"=0.0, "Value"=0.0}, "Parameter name"=w380, "Value"=w379, "Time (ms)"=w378) -> (w360:T11)
                  n132 = To Variant(anything=w360) -> (Variant=w374:variant)
                  n133 = Bundle By Name(cluster=T10 {"Data"=variant, "Command"=enum."Plotter_Update"} ("element"), "Data"=w374) -> (w366:T10)
                  n134 = Enqueue Element(queue=w376, element=w366, error in (no error)=w377) -> (error out=w373:errorcluster)  [unwired: 1 in, 2 out]
                  n135 = To Variant(anything=w360) -> (Variant=w364:variant)
                  n136 = Bundle By Name(cluster=T10 {"Data"=variant, "Command"=enum."UI Indicators Update"} ("element"), "Data"=w364) -> (w363:T10)
                  n137 = case shown="True" w372 {
                    tunnel: w373 -> [w394 w398]
                    tunnel: [w394 w396] -> w371
                    tunnel: w368 -> [_ w397]
                    tunnel: w363 -> [_ w395]
                    frame False {
                    }
                    frame True {
                      n138 = Enqueue Element(queue=w397, element=w395, error in (no error)=w398) -> (error out=w396:errorcluster)  [unwired: 1 in, 2 out]
                    }
                  }
                  n139 = To Variant(anything=w360) -> (Variant=w361:variant)
                  n140 = Bundle By Name(cluster=T10 {"Data"=variant, "Command"=enum."3D Viewer Update"} ("element"), "Data"=w361) -> (w359:T10)
                  n141 = case shown="True" w370 {
                    tunnel: w371 -> [w389 w393]
                    tunnel: [w389 w390] -> w369
                    tunnel: w367 -> [_ w392]
                    tunnel: w359 -> [_ w391]
                    frame False {
                    }
                    frame True {
                      n142 = Enqueue Element(queue=w392, element=w391, error in (no error)=w393) -> (error out=w390:errorcluster)  [unwired: 1 in, 2 out]
                    }
                  }
                }
              }
              frame 34 {
                w403 = FALSE ("Initialize ?")
                # "IMU_X_ACCEL_PROCESSED\nIMU_X_GYRO_PROCESSED"
                n143 = Unbundle By Name(w412) -> ("MPU_Stick_Queues.3D View Updater"=w409:refnum<queue>, "MPU_Stick_Queues.Plot Updater"=w408:refnum<queue>, "MPU_Stick_Queues.UI Indicators Updater"=w407:refnum<queue>)
                n144 = call "MPU_Stick_Event_Counter.vi"("Initialize ?"=w403, "error in (no error)"=w406, "Event Name"="MP_PITCH_ACCEL_3D_Viewer_Update") -> ("error out"=w405:errorcluster, "Event occured"=w399:bool)  [unwired: 6 in, 1 out]
                n145 = call "MPU_Stick_Event_Counter.vi"("Initialize ?"=w403, "error in (no error)"=w405, "Event Name"="MP_PITCH_ACCEL_UI_Indicator_Update") -> ("error out"=w404:errorcluster, "Event occured"=w400:bool)  [unwired: 6 in, 1 out]
                n146 = for {
                  shift-right: [w443] -> w413
                  shift-left: w415 -> [w445]
                  tunnel: string[] ["PITCH_ACCEL"] -> [w437] mode=indexing
                  shift-right: [w426] -> w410
                  shift-left: w404 -> [w444]
                  tunnel: string[] ["MPU_STICK:MP_PITCH_ACCEL:MP_PITCH_ACCEL"] -> [w440] mode=indexing
                  tunnel: w409 -> [w424]
                  tunnel: w408 -> [w433]
                  tunnel: w407 -> [w425]
                  tunnel: w400 -> [w429]
                  tunnel: w399 -> [w427]
                  n147 = call "ADCP_read_parameter.vi"("error in (no error)"=w444, "Parameter Name"=w440, "ADCP In"=w445) -> ("error out"=w434:errorcluster, "Parameter Value"=w442:string, "Data Packet out"=w441:T14, "ADCP out"=w443:refnum<class "ADCP.lvclass">)  [unwired: 5 in]
                  n148 = Unbundle By Name(w441) -> ("Last Rx Time"=w439:u32)
                  n149 = Fract/Exp String To Number(string=w442) -> (number=w436:dbl)  [unwired: 3 in, 1 out]
                  n150 = To Double Precision Float(number=w439) -> (double precision float=w435:dbl)
                  n151 = Bundle By Name(cluster=T11 {"Parameter name"="", "Time (ms)"=0.0, "Value"=0.0}, "Parameter name"=w437, "Value"=w436, "Time (ms)"=w435) -> (w417:T11)
                  n152 = To Variant(anything=w417) -> (Variant=w431:variant)
                  n153 = Bundle By Name(cluster=T10 {"Data"=variant, "Command"=enum."Plotter_Update"} ("element"), "Data"=w431) -> (w423:T10)
                  n154 = Enqueue Element(queue=w433, element=w423, error in (no error)=w434) -> (error out=w430:errorcluster)  [unwired: 1 in, 2 out]
                  n155 = To Variant(anything=w417) -> (Variant=w421:variant)
                  n156 = Bundle By Name(cluster=T10 {"Data"=variant, "Command"=enum."UI Indicators Update"} ("element"), "Data"=w421) -> (w420:T10)
                  n157 = case shown="True" w429 {
                    tunnel: w430 -> [w451 w455]
                    tunnel: [w451 w453] -> w428
                    tunnel: w425 -> [_ w454]
                    tunnel: w420 -> [_ w452]
                    frame False {
                    }
                    frame True {
                      n158 = Enqueue Element(queue=w454, element=w452, error in (no error)=w455) -> (error out=w453:errorcluster)  [unwired: 1 in, 2 out]
                    }
                  }
                  n159 = To Variant(anything=w417) -> (Variant=w418:variant)
                  n160 = Bundle By Name(cluster=T10 {"Data"=variant, "Command"=enum."3D Viewer Update"} ("element"), "Data"=w418) -> (w416:T10)
                  n161 = case shown="True" w427 {
                    tunnel: w428 -> [w446 w450]
                    tunnel: [w446 w447] -> w426
                    tunnel: w424 -> [_ w449]
                    tunnel: w416 -> [_ w448]
                    frame False {
                    }
                    frame True {
                      n162 = Enqueue Element(queue=w449, element=w448, error in (no error)=w450) -> (error out=w447:errorcluster)  [unwired: 1 in, 2 out]
                    }
                  }
                }
              }
              frame 35 {
                w460 = FALSE ("Initialize ?")
                # "IMU_X_ACCEL_PROCESSED\nIMU_X_GYRO_PROCESSED"
                n163 = Unbundle By Name(w469) -> ("MPU_Stick_Queues.3D View Updater"=w466:refnum<queue>, "MPU_Stick_Queues.Plot Updater"=w465:refnum<queue>, "MPU_Stick_Queues.UI Indicators Updater"=w464:refnum<queue>)
                n164 = call "MPU_Stick_Event_Counter.vi"("Initialize ?"=w460, "error in (no error)"=w463, "Event Name"="MP_PITCH_GYRO_3D_Viewer_Update") -> ("error out"=w462:errorcluster, "Event occured"=w456:bool)  [unwired: 6 in, 1 out]
                n165 = call "MPU_Stick_Event_Counter.vi"("Initialize ?"=w460, "error in (no error)"=w462, "Event Name"="MP_PITCH_GYRO_UI_Indicator_Update") -> ("error out"=w461:errorcluster, "Event occured"=w457:bool)  [unwired: 6 in, 1 out]
                n166 = for {
                  shift-right: [w500] -> w470
                  shift-left: w472 -> [w502]
                  tunnel: string[] ["PITCH_GYRO"] -> [w494] mode=indexing
                  shift-right: [w483] -> w467
                  shift-left: w461 -> [w501]
                  tunnel: string[] ["MPU_STICK:MP_PITCH_GYRO:MP_PITCH_GYRO"] -> [w497] mode=indexing
                  tunnel: w466 -> [w481]
                  tunnel: w465 -> [w490]
                  tunnel: w464 -> [w482]
                  tunnel: w457 -> [w486]
                  tunnel: w456 -> [w484]
                  n167 = call "ADCP_read_parameter.vi"("error in (no error)"=w501, "Parameter Name"=w497, "ADCP In"=w502) -> ("error out"=w491:errorcluster, "Parameter Value"=w499:string, "Data Packet out"=w498:T14, "ADCP out"=w500:refnum<class "ADCP.lvclass">)  [unwired: 5 in]
                  n168 = Unbundle By Name(w498) -> ("Last Rx Time"=w496:u32)
                  n169 = Fract/Exp String To Number(string=w499) -> (number=w493:dbl)  [unwired: 3 in, 1 out]
                  n170 = To Double Precision Float(number=w496) -> (double precision float=w492:dbl)
                  n171 = Bundle By Name(cluster=T11 {"Parameter name"="", "Time (ms)"=0.0, "Value"=0.0}, "Parameter name"=w494, "Value"=w493, "Time (ms)"=w492) -> (w474:T11)
                  n172 = To Variant(anything=w474) -> (Variant=w488:variant)
                  n173 = Bundle By Name(cluster=T10 {"Data"=variant, "Command"=enum."Plotter_Update"} ("element"), "Data"=w488) -> (w480:T10)
                  n174 = Enqueue Element(queue=w490, element=w480, error in (no error)=w491) -> (error out=w487:errorcluster)  [unwired: 1 in, 2 out]
                  n175 = To Variant(anything=w474) -> (Variant=w478:variant)
                  n176 = Bundle By Name(cluster=T10 {"Data"=variant, "Command"=enum."UI Indicators Update"} ("element"), "Data"=w478) -> (w477:T10)
                  n177 = case shown="True" w486 {
                    tunnel: w487 -> [w508 w512]
                    tunnel: [w508 w510] -> w485
                    tunnel: w482 -> [_ w511]
                    tunnel: w477 -> [_ w509]
                    frame False {
                    }
                    frame True {
                      n178 = Enqueue Element(queue=w511, element=w509, error in (no error)=w512) -> (error out=w510:errorcluster)  [unwired: 1 in, 2 out]
                    }
                  }
                  n179 = To Variant(anything=w474) -> (Variant=w475:variant)
                  n180 = Bundle By Name(cluster=T10 {"Data"=variant, "Command"=enum."3D Viewer Update"} ("element"), "Data"=w475) -> (w473:T10)
                  n181 = case shown="True" w484 {
                    tunnel: w485 -> [w503 w507]
                    tunnel: [w503 w504] -> w483
                    tunnel: w481 -> [_ w506]
                    tunnel: w473 -> [_ w505]
                    frame False {
                    }
                    frame True {
                      n182 = Enqueue Element(queue=w506, element=w505, error in (no error)=w507) -> (error out=w504:errorcluster)  [unwired: 1 in, 2 out]
                    }
                  }
                }
              }
              frame 36 {
                w517 = FALSE ("Initialize ?")
                # "IMU_X_ACCEL_PROCESSED\nIMU_X_GYRO_PROCESSED"
                n183 = Unbundle By Name(w526) -> ("MPU_Stick_Queues.3D View Updater"=w523:refnum<queue>, "MPU_Stick_Queues.Plot Updater"=w522:refnum<queue>, "MPU_Stick_Queues.UI Indicators Updater"=w521:refnum<queue>)
                n184 = call "MPU_Stick_Event_Counter.vi"("Initialize ?"=w517, "error in (no error)"=w520, "Event Name"="MP_PITCH_FILTER_3D_Viewer_Update") -> ("error out"=w519:errorcluster, "Event occured"=w513:bool)  [unwired: 6 in, 1 out]
                n185 = call "MPU_Stick_Event_Counter.vi"("Initialize ?"=w517, "error in (no error)"=w519, "Event Name"="MP_PITCH_FILTER_UI_Indicator_Update") -> ("error out"=w518:errorcluster, "Event occured"=w514:bool)  [unwired: 6 in, 1 out]
                n186 = for {
                  shift-right: [w557] -> w527
                  shift-left: w529 -> [w559]
                  tunnel: string[] ["PITCH_COMP_FILTER"] -> [w551] mode=indexing
                  shift-right: [w540] -> w524
                  shift-left: w518 -> [w558]
                  tunnel: string[] ["MPU_STICK:MP_PITCH_FILTER:MP_PITCH_FILTER"] -> [w554] mode=indexing
                  tunnel: w523 -> [w538]
                  tunnel: w522 -> [w547]
                  tunnel: w521 -> [w539]
                  tunnel: w514 -> [w543]
                  tunnel: w513 -> [w541]
                  n187 = call "ADCP_read_parameter.vi"("error in (no error)"=w558, "Parameter Name"=w554, "ADCP In"=w559) -> ("error out"=w548:errorcluster, "Parameter Value"=w556:string, "Data Packet out"=w555:T14, "ADCP out"=w557:refnum<class "ADCP.lvclass">)  [unwired: 5 in]
                  n188 = Unbundle By Name(w555) -> ("Last Rx Time"=w553:u32)
                  n189 = Fract/Exp String To Number(string=w556) -> (number=w550:dbl)  [unwired: 3 in, 1 out]
                  n190 = To Double Precision Float(number=w553) -> (double precision float=w549:dbl)
                  n191 = Bundle By Name(cluster=T11 {"Parameter name"="", "Time (ms)"=0.0, "Value"=0.0}, "Parameter name"=w551, "Value"=w550, "Time (ms)"=w549) -> (w531:T11)
                  n192 = To Variant(anything=w531) -> (Variant=w545:variant)
                  n193 = Bundle By Name(cluster=T10 {"Data"=variant, "Command"=enum."Plotter_Update"} ("element"), "Data"=w545) -> (w537:T10)
                  n194 = Enqueue Element(queue=w547, element=w537, error in (no error)=w548) -> (error out=w544:errorcluster)  [unwired: 1 in, 2 out]
                  n195 = To Variant(anything=w531) -> (Variant=w535:variant)
                  n196 = Bundle By Name(cluster=T10 {"Data"=variant, "Command"=enum."UI Indicators Update"} ("element"), "Data"=w535) -> (w534:T10)
                  n197 = case shown="True" w543 {
                    tunnel: w544 -> [w565 w569]
                    tunnel: [w565 w567] -> w542
                    tunnel: w539 -> [_ w568]
                    tunnel: w534 -> [_ w566]
                    frame False {
                    }
                    frame True {
                      n198 = Enqueue Element(queue=w568, element=w566, error in (no error)=w569) -> (error out=w567:errorcluster)  [unwired: 1 in, 2 out]
                    }
                  }
                  n199 = To Variant(anything=w531) -> (Variant=w532:variant)
                  n200 = Bundle By Name(cluster=T10 {"Data"=variant, "Command"=enum."3D Viewer Update"} ("element"), "Data"=w532) -> (w530:T10)
                  n201 = case shown="True" w541 {
                    tunnel: w542 -> [w560 w564]
                    tunnel: [w560 w561] -> w540
                    tunnel: w538 -> [_ w563]
                    tunnel: w530 -> [_ w562]
                    frame False {
                    }
                    frame True {
                      n202 = Enqueue Element(queue=w563, element=w562, error in (no error)=w564) -> (error out=w561:errorcluster)  [unwired: 1 in, 2 out]
                    }
                  }
                }
              }
              frame 37 {
                w574 = FALSE ("Initialize ?")
                # "IMU_X_ACCEL_PROCESSED\nIMU_X_GYRO_PROCESSED"
                n203 = Unbundle By Name(w583) -> ("MPU_Stick_Queues.3D View Updater"=w580:refnum<queue>, "MPU_Stick_Queues.Plot Updater"=w579:refnum<queue>, "MPU_Stick_Queues.UI Indicators Updater"=w578:refnum<queue>)
                n204 = call "MPU_Stick_Event_Counter.vi"("Initialize ?"=w574, "error in (no error)"=w577, "Event Name"="MP_YAW_ACCEL_3D_Viewer_Update") -> ("error out"=w576:errorcluster, "Event occured"=w570:bool)  [unwired: 6 in, 1 out]
                n205 = call "MPU_Stick_Event_Counter.vi"("Initialize ?"=w574, "error in (no error)"=w576, "Event Name"="MP_YAW_ACCEL_UI_Indicator_Update") -> ("error out"=w575:errorcluster, "Event occured"=w571:bool)  [unwired: 6 in, 1 out]
                n206 = for {
                  shift-right: [w614] -> w584
                  shift-left: w586 -> [w616]
                  tunnel: string[] ["YAW_ACCEL"] -> [w608] mode=indexing
                  shift-right: [w597] -> w581
                  shift-left: w575 -> [w615]
                  tunnel: string[] ["MPU_STICK:MP_YAW_ACCEL:MP_YAW_ACCEL"] -> [w611] mode=indexing
                  tunnel: w580 -> [w595]
                  tunnel: w579 -> [w604]
                  tunnel: w578 -> [w596]
                  tunnel: w571 -> [w600]
                  tunnel: w570 -> [w598]
                  n207 = call "ADCP_read_parameter.vi"("error in (no error)"=w615, "Parameter Name"=w611, "ADCP In"=w616) -> ("error out"=w605:errorcluster, "Parameter Value"=w613:string, "Data Packet out"=w612:T14, "ADCP out"=w614:refnum<class "ADCP.lvclass">)  [unwired: 5 in]
                  n208 = Unbundle By Name(w612) -> ("Last Rx Time"=w610:u32)
                  n209 = Fract/Exp String To Number(string=w613) -> (number=w607:dbl)  [unwired: 3 in, 1 out]
                  n210 = To Double Precision Float(number=w610) -> (double precision float=w606:dbl)
                  n211 = Bundle By Name(cluster=T11 {"Parameter name"="", "Time (ms)"=0.0, "Value"=0.0}, "Parameter name"=w608, "Value"=w607, "Time (ms)"=w606) -> (w588:T11)
                  n212 = To Variant(anything=w588) -> (Variant=w602:variant)
                  n213 = Bundle By Name(cluster=T10 {"Data"=variant, "Command"=enum."Plotter_Update"} ("element"), "Data"=w602) -> (w594:T10)
                  n214 = Enqueue Element(queue=w604, element=w594, error in (no error)=w605) -> (error out=w601:errorcluster)  [unwired: 1 in, 2 out]
                  n215 = To Variant(anything=w588) -> (Variant=w592:variant)
                  n216 = Bundle By Name(cluster=T10 {"Data"=variant, "Command"=enum."UI Indicators Update"} ("element"), "Data"=w592) -> (w591:T10)
                  n217 = case shown="True" w600 {
                    tunnel: w601 -> [w622 w626]
                    tunnel: [w622 w624] -> w599
                    tunnel: w596 -> [_ w625]
                    tunnel: w591 -> [_ w623]
                    frame False {
                    }
                    frame True {
                      n218 = Enqueue Element(queue=w625, element=w623, error in (no error)=w626) -> (error out=w624:errorcluster)  [unwired: 1 in, 2 out]
                    }
                  }
                  n219 = To Variant(anything=w588) -> (Variant=w589:variant)
                  n220 = Bundle By Name(cluster=T10 {"Data"=variant, "Command"=enum."3D Viewer Update"} ("element"), "Data"=w589) -> (w587:T10)
                  n221 = case shown="True" w598 {
                    tunnel: w599 -> [w617 w621]
                    tunnel: [w617 w618] -> w597
                    tunnel: w595 -> [_ w620]
                    tunnel: w587 -> [_ w619]
                    frame False {
                    }
                    frame True {
                      n222 = Enqueue Element(queue=w620, element=w619, error in (no error)=w621) -> (error out=w618:errorcluster)  [unwired: 1 in, 2 out]
                    }
                  }
                }
              }
              frame 38 {
                w631 = FALSE ("Initialize ?")
                # "IMU_X_ACCEL_PROCESSED\nIMU_X_GYRO_PROCESSED"
                n223 = Unbundle By Name(w640) -> ("MPU_Stick_Queues.3D View Updater"=w637:refnum<queue>, "MPU_Stick_Queues.Plot Updater"=w636:refnum<queue>, "MPU_Stick_Queues.UI Indicators Updater"=w635:refnum<queue>)
                n224 = call "MPU_Stick_Event_Counter.vi"("Initialize ?"=w631, "error in (no error)"=w634, "Event Name"="MP_YAW_GYRO_3D_Viewer_Update") -> ("error out"=w633:errorcluster, "Event occured"=w627:bool)  [unwired: 6 in, 1 out]
                n225 = call "MPU_Stick_Event_Counter.vi"("Initialize ?"=w631, "error in (no error)"=w633, "Event Name"="MP_YAW_GYRO_UI_Indicator_Update") -> ("error out"=w632:errorcluster, "Event occured"=w628:bool)  [unwired: 6 in, 1 out]
                n226 = for {
                  shift-right: [w671] -> w641
                  shift-left: w643 -> [w673]
                  tunnel: string[] ["YAW_GYRO"] -> [w665] mode=indexing
                  shift-right: [w654] -> w638
                  shift-left: w632 -> [w672]
                  tunnel: string[] ["MPU_STICK:MP_YAW_GYRO:MP_YAW_GYRO"] -> [w668] mode=indexing
                  tunnel: w637 -> [w652]
                  tunnel: w636 -> [w661]
                  tunnel: w635 -> [w653]
                  tunnel: w628 -> [w657]
                  tunnel: w627 -> [w655]
                  n227 = call "ADCP_read_parameter.vi"("error in (no error)"=w672, "Parameter Name"=w668, "ADCP In"=w673) -> ("error out"=w662:errorcluster, "Parameter Value"=w670:string, "Data Packet out"=w669:T14, "ADCP out"=w671:refnum<class "ADCP.lvclass">)  [unwired: 5 in]
                  n228 = Unbundle By Name(w669) -> ("Last Rx Time"=w667:u32)
                  n229 = Fract/Exp String To Number(string=w670) -> (number=w664:dbl)  [unwired: 3 in, 1 out]
                  n230 = To Double Precision Float(number=w667) -> (double precision float=w663:dbl)
                  n231 = Bundle By Name(cluster=T11 {"Parameter name"="", "Time (ms)"=0.0, "Value"=0.0}, "Parameter name"=w665, "Value"=w664, "Time (ms)"=w663) -> (w645:T11)
                  n232 = To Variant(anything=w645) -> (Variant=w659:variant)
                  n233 = Bundle By Name(cluster=T10 {"Data"=variant, "Command"=enum."Plotter_Update"} ("element"), "Data"=w659) -> (w651:T10)
                  n234 = Enqueue Element(queue=w661, element=w651, error in (no error)=w662) -> (error out=w658:errorcluster)  [unwired: 1 in, 2 out]
                  n235 = To Variant(anything=w645) -> (Variant=w649:variant)
                  n236 = Bundle By Name(cluster=T10 {"Data"=variant, "Command"=enum."UI Indicators Update"} ("element"), "Data"=w649) -> (w648:T10)
                  n237 = case shown="True" w657 {
                    tunnel: w658 -> [w679 w683]
                    tunnel: [w679 w681] -> w656
                    tunnel: w653 -> [_ w682]
                    tunnel: w648 -> [_ w680]
                    frame False {
                    }
                    frame True {
                      n238 = Enqueue Element(queue=w682, element=w680, error in (no error)=w683) -> (error out=w681:errorcluster)  [unwired: 1 in, 2 out]
                    }
                  }
                  n239 = To Variant(anything=w645) -> (Variant=w646:variant)
                  n240 = Bundle By Name(cluster=T10 {"Data"=variant, "Command"=enum."3D Viewer Update"} ("element"), "Data"=w646) -> (w644:T10)
                  n241 = case shown="True" w655 {
                    tunnel: w656 -> [w674 w678]
                    tunnel: [w674 w675] -> w654
                    tunnel: w652 -> [_ w677]
                    tunnel: w644 -> [_ w676]
                    frame False {
                    }
                    frame True {
                      n242 = Enqueue Element(queue=w677, element=w676, error in (no error)=w678) -> (error out=w675:errorcluster)  [unwired: 1 in, 2 out]
                    }
                  }
                }
              }
              frame 39 {
                w688 = FALSE ("Initialize ?")
                # "IMU_X_ACCEL_PROCESSED\nIMU_X_GYRO_PROCESSED"
                n243 = Unbundle By Name(w697) -> ("MPU_Stick_Queues.3D View Updater"=w694:refnum<queue>, "MPU_Stick_Queues.Plot Updater"=w693:refnum<queue>, "MPU_Stick_Queues.UI Indicators Updater"=w692:refnum<queue>)
                n244 = call "MPU_Stick_Event_Counter.vi"("Initialize ?"=w688, "error in (no error)"=w691, "Event Name"="MP_YAW_FILTER_3D_Viewer_Update") -> ("error out"=w690:errorcluster, "Event occured"=w684:bool)  [unwired: 6 in, 1 out]
                n245 = call "MPU_Stick_Event_Counter.vi"("Initialize ?"=w688, "error in (no error)"=w690, "Event Name"="MP_YAW_FILTER_UI_Indicator_Update") -> ("error out"=w689:errorcluster, "Event occured"=w685:bool)  [unwired: 6 in, 1 out]
                n246 = for {
                  shift-right: [w728] -> w698
                  shift-left: w700 -> [w730]
                  tunnel: string[] ["YAW_COMP_FILTER"] -> [w722] mode=indexing
                  shift-right: [w711] -> w695
                  shift-left: w689 -> [w729]
                  tunnel: string[] ["MPU_STICK:MP_YAW_FILTER:MP_YAW_FILTER"] -> [w725] mode=indexing
                  tunnel: w694 -> [w709]
                  tunnel: w693 -> [w718]
                  tunnel: w692 -> [w710]
                  tunnel: w685 -> [w714]
                  tunnel: w684 -> [w712]
                  n247 = call "ADCP_read_parameter.vi"("error in (no error)"=w729, "Parameter Name"=w725, "ADCP In"=w730) -> ("error out"=w719:errorcluster, "Parameter Value"=w727:string, "Data Packet out"=w726:T14, "ADCP out"=w728:refnum<class "ADCP.lvclass">)  [unwired: 5 in]
                  n248 = Unbundle By Name(w726) -> ("Last Rx Time"=w724:u32)
                  n249 = Fract/Exp String To Number(string=w727) -> (number=w721:dbl)  [unwired: 3 in, 1 out]
                  n250 = To Double Precision Float(number=w724) -> (double precision float=w720:dbl)
                  n251 = Bundle By Name(cluster=T11 {"Parameter name"="", "Time (ms)"=0.0, "Value"=0.0}, "Parameter name"=w722, "Value"=w721, "Time (ms)"=w720) -> (w702:T11)
                  n252 = To Variant(anything=w702) -> (Variant=w716:variant)
                  n253 = Bundle By Name(cluster=T10 {"Data"=variant, "Command"=enum."Plotter_Update"} ("element"), "Data"=w716) -> (w708:T10)
                  n254 = Enqueue Element(queue=w718, element=w708, error in (no error)=w719) -> (error out=w715:errorcluster)  [unwired: 1 in, 2 out]
                  n255 = To Variant(anything=w702) -> (Variant=w706:variant)
                  n256 = Bundle By Name(cluster=T10 {"Data"=variant, "Command"=enum."UI Indicators Update"} ("element"), "Data"=w706) -> (w705:T10)
                  n257 = case shown="True" w714 {
                    tunnel: w715 -> [w736 w740]
                    tunnel: [w736 w738] -> w713
                    tunnel: w710 -> [_ w739]
                    tunnel: w705 -> [_ w737]
                    frame False {
                    }
                    frame True {
                      n258 = Enqueue Element(queue=w739, element=w737, error in (no error)=w740) -> (error out=w738:errorcluster)  [unwired: 1 in, 2 out]
                    }
                  }
                  n259 = To Variant(anything=w702) -> (Variant=w703:variant)
                  n260 = Bundle By Name(cluster=T10 {"Data"=variant, "Command"=enum."3D Viewer Update"} ("element"), "Data"=w703) -> (w701:T10)
                  n261 = case shown="True" w712 {
                    tunnel: w713 -> [w731 w735]
                    tunnel: [w731 w732] -> w711
                    tunnel: w709 -> [_ w734]
                    tunnel: w701 -> [_ w733]
                    frame False {
                    }
                    frame True {
                      n262 = Enqueue Element(queue=w734, element=w733, error in (no error)=w735) -> (error out=w732:errorcluster)  [unwired: 1 in, 2 out]
                    }
                  }
                }
              }
              frame 41 {
                w745 = FALSE ("Initialize ?")
                # "IMU_X_ACCEL_PROCESSED\nIMU_X_GYRO_PROCESSED"
                n263 = Unbundle By Name(w754) -> ("MPU_Stick_Queues.3D View Updater"=w751:refnum<queue>, "MPU_Stick_Queues.Plot Updater"=w750:refnum<queue>, "MPU_Stick_Queues.UI Indicators Updater"=w749:refnum<queue>)
                n264 = call "MPU_Stick_Event_Counter.vi"("Initialize ?"=w745, "error in (no error)"=w748, "Event Name"="MD_OUTPUT_3D_Viewer_Update") -> ("error out"=w747:errorcluster, "Event occured"=w741:bool)  [unwired: 6 in, 1 out]
                n265 = call "MPU_Stick_Event_Counter.vi"("Initialize ?"=w745, "error in (no error)"=w747, "Event Name"="MD_OUTPUT_UI_Indicator_Update") -> ("error out"=w746:errorcluster, "Event occured"=w742:bool)  [unwired: 6 in, 1 out]
                n266 = for {
                  shift-right: [w785] -> w755
                  shift-left: w757 -> [w787]
                  tunnel: string[] ["MD_OUTPUT_ACCEL_X", "MD_OUTPUT_ACCEL_Y", "MD_OUTPUT_ACCEL_Z", "MD_OUTPUT_GYRO_X", "MD_OUTPUT_GYRO_Y", "MD_OUTPUT_GYRO_Z", "MD_OUTPUT_ROLL", "MD_OUTPUT_PITCH", "MD_OUTPUT_YAW"] -> [w779] mode=indexing
                  shift-right: [w768] -> w752
                  shift-left: w746 -> [w786]
                  tunnel: string[] ["MPU_STICK:MD_OUTPUT:MD_OUTPUT_ACCEL_X", "MPU_STICK:MD_OUTPUT:MD_OUTPUT_ACCEL_Y", "MPU_STICK:MD_OUTPUT:MD_OUTPUT_ACCEL_Z", "MPU_STICK:MD_OUTPUT:MD_OUTPUT_GYRO_X", "MPU_STICK:MD_OUTPUT:MD_OUTPUT_GYRO_Y", "MPU_STICK:MD_OUTPUT:MD_OUTPUT_GYRO_Z", "MPU_STICK:MD_OUTPUT:MD_OUTPUT_ROLL", "MPU_STICK:MD_OUTPUT:MD_OUTPUT_PITCH", "MPU_STICK:MD_OUTPUT:MD_OUTPUT_YAW"] -> [w782] mode=indexing
                  tunnel: w751 -> [w766]
                  tunnel: w750 -> [w775]
                  tunnel: w749 -> [w767]
                  tunnel: w742 -> [w771]
                  tunnel: w741 -> [w769]
                  n267 = call "ADCP_read_parameter.vi"("error in (no error)"=w786, "Parameter Name"=w782, "ADCP In"=w787) -> ("error out"=w776:errorcluster, "Parameter Value"=w784:string, "Data Packet out"=w783:T14, "ADCP out"=w785:refnum<class "ADCP.lvclass">)  [unwired: 5 in]
                  n268 = Unbundle By Name(w783) -> ("Last Rx Time"=w781:u32)
                  n269 = Fract/Exp String To Number(string=w784) -> (number=w778:dbl)  [unwired: 3 in, 1 out]
                  n270 = To Double Precision Float(number=w781) -> (double precision float=w777:dbl)
                  n271 = Bundle By Name(cluster=T11 {"Parameter name"="", "Time (ms)"=0.0, "Value"=0.0}, "Parameter name"=w779, "Value"=w778, "Time (ms)"=w777) -> (w759:T11)
                  n272 = To Variant(anything=w759) -> (Variant=w773:variant)
                  n273 = Bundle By Name(cluster=T10 {"Data"=variant, "Command"=enum."Plotter_Update"} ("element"), "Data"=w773) -> (w765:T10)
                  n274 = disable-structure shown="Disabled" {
                    disable-tunnel: w776 -> [w791 w792]
                    disable-tunnel: w775 -> [w790 _]
                    disable-tunnel: [w789 w792] -> w772
                    disable-tunnel: w765 -> [w788 _]
                    frame Disabled {
                      n275 = Enqueue Element(queue=w790, element=w788, error in (no error)=w791) -> (error out=w789:errorcluster)  [unwired: 1 in, 2 out]
                    }
                    frame Enabled {
                    }
                  }
                  n276 = To Variant(anything=w759) -> (Variant=w763:variant)
                  n277 = Bundle By Name(cluster=T10 {"Data"=variant, "Command"=enum."UI Indicators Update"} ("element"), "Data"=w763) -> (w762:T10)
                  n278 = case shown="True" w771 {
                    tunnel: w772 -> [w798 w802]
                    tunnel: [w798 w800] -> w770
                    tunnel: w767 -> [_ w801]
                    tunnel: w762 -> [_ w799]
                    frame False {
                    }
                    frame True {
                      n279 = Enqueue Element(queue=w801, element=w799, error in (no error)=w802) -> (error out=w800:errorcluster)  [unwired: 1 in, 2 out]
                    }
                  }
                  n280 = To Variant(anything=w759) -> (Variant=w760:variant)
                  n281 = Bundle By Name(cluster=T10 {"Data"=variant, "Command"=enum."3D Viewer Update"} ("element"), "Data"=w760) -> (w758:T10)
                  n282 = case shown="True" w769 {
                    tunnel: w770 -> [w793 w797]
                    tunnel: [w793 w794] -> w768
                    tunnel: w766 -> [_ w796]
                    tunnel: w758 -> [_ w795]
                    frame False {
                    }
                    frame True {
                      n283 = Enqueue Element(queue=w796, element=w795, error in (no error)=w797) -> (error out=w794:errorcluster)  [unwired: 1 in, 2 out]
                    }
                  }
                }
              }
            }
          }
          frame Disabled {
          }
        }
        n284 = property class="LVClassControl (strict)"(reference=w43, "Value"=w39) -> ()  [unwired: 1 in, 2 out]
      }
    }
  }
